vi "Interface Browser.vi"(5 "Caller Window Bounds":T1, 7 "Name (\"\" to Use Uuid)":string=".interface-browser", 10 "Init State (\"Macro: Initialize\")":string="Macro: Initialize") -> ()   [LabVIEW 2017]
uses:
  <vilib>/Utility/miscctls.llb/LVRectTypeDef.ctl
  Def-FilterOption.ctl
  <vilib>/Utility/miscctls.llb/LVPoint32TypeDef.ctl
  Def-TreeData.ctl
  <vilib>/Utility/miscctls.llb/LVPointTypeDef.ctl
  AdvanceAPI/CSM - Revert Arguments-Safe String.vi
  AdvanceAPI/CSM - Break Down Multiple States String.vi
  AdvanceAPI/CSM - Compact Multiple States.vi
  AdvanceAPI/CSM - Make String Arguments Safe.vi
  AdvanceAPI/CSM - Keywords.vi
  _Polymophic/Add State(s) to Queue By BOOL(Element).vi
  _csmHelper/API/Destroy.vi
  _csmHelper/API/Stop Undo.vi
  _csmHelper/API/Open Block Diagram.vi
  _csmHelper/API/Connect Paired Tunnels.vi
  _csmHelper/API/Add State Frame.vi
  _csmHelper/API/Start Undo.vi
  _csmHelper/API/Create From VI Reference.vi
  _csmHelper/API/Open Front Panel.vi
  _Polymophic/CSM - Filter Duplicated Lines.vi
  Communicable State Machine.lvlib
  _ui/csm-ui-support.lvlib
  _csmHelper/API with lvcsm Support/CSM-Helper API with lvcsm Support.lvlib
  _interfacebrowser/interfacebrowser.lvlib
  _csmHelper/CSM-Helper.lvclass
  _csmHelper/lvcsmFile/lvcsm File Support.lvlib
  _Shared/CSM Shared.lvlib
panel:
  in  "Option:All-CSM-VIs":bool
  in  "Scan Project":bool
  in  "Refresh":bool
  in  "Fast Forward":bool
  in  "Fast Reverse":bool
  in  "Skip to Beginning":bool
  in  "Skip to End":bool
  in  "Stop":bool
  in  "Play":bool
  in  "Open":bool
  in  "Option:Online Only":bool
  in  "Refresh lvcsm Cache":bool
  in  "Filter":string
  in  "FilterOption":T2
  in  "Reset Filter":bool
  in  "MainTree":string[](tree)
  in  "Option:Sync Filter On States":bool
  in  "Zoom Factor":dbl(slide)=0.1 min=0.1 max=1.0 step=0.001 scale=0.1..1.0
  in  "Interface-Filter":enum16{"API-Only", "UserDef States", "All"}(ring)=enum."UserDef States"
  in  "CSM-States":i32[](listbox) caption="Interface"
  in  "CSM-Status":i32[](listbox) caption="Status"
  out "StateInfo@Image":string
  out "Preview":picture
  out "String":string
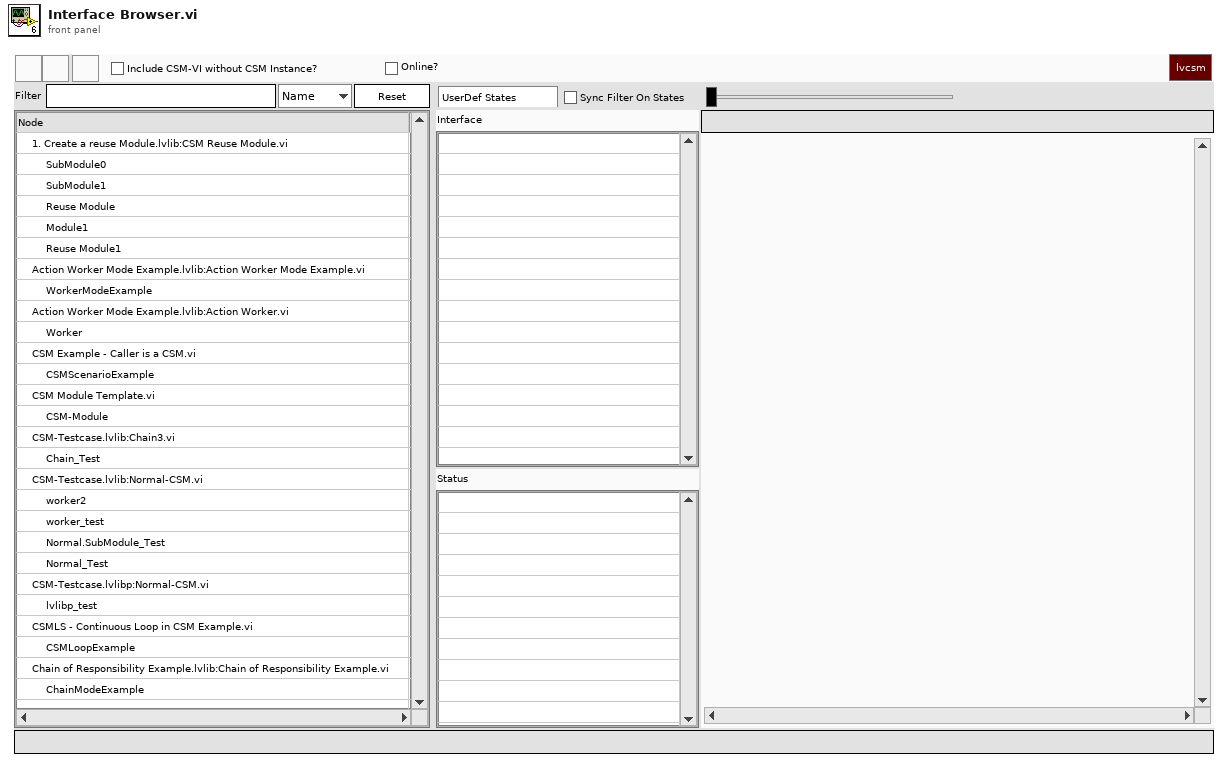
[diagram p1: front panel]
types:
  T1 = typedef "LVRectTypeDef.ctl" = cluster{"Left":i16, "Top":i16, "Right":i16, "Bottom":i16}
  T2 = typedef "Def-FilterOption.ctl" = enum16{"Name", "State"}
  T3 = enum32{"Invalid", "Standard", "Closed", "Hidden", "Minimized", "Maximized"}
  T4 = enum32{"invalid app kind", "Development System", "Run Time System", "Student Edition", "Embedded LabVIEW", "Evaluation", "Custom"}
  T5 = typedef "LVPointTypeDef.ctl" = cluster{"Horizontal":i16, "Vertical":i16}
  T6 = cluster{"Opton:All-CSM-VIs":bool, "Option:Online Only":bool}
  T7 = typedef "Communicable State Machine.lvlib/_CSM_Response Source Message.ctl" = cluster{"‘State":string, "’Arguments":string, "’Error":errorcluster}
  T8 = cluster{"Current VI Reference":refnum<vi>, "Close Panel on Exit?":bool}
  T9 = typedef "Def-TreeData.ctl" = cluster{"Type":string[], "Table":string[][]}
  T10 = cluster{"Core":cluster{"Current VI Reference":refnum<vi>, "Close Panel on Exit?":bool}, "BD-IMG":picture, "Tree":T9}
  T11 = typedef "LVPoint32TypeDef.ctl" = cluster{"Horizontal":i32, "Vertical":i32}
  T12 = cluster{"your data":bool, "PreviewMouseDown":bool, "PreviewMouseDownCoords":T11, "PreviewMouseDownOrigin":T11}
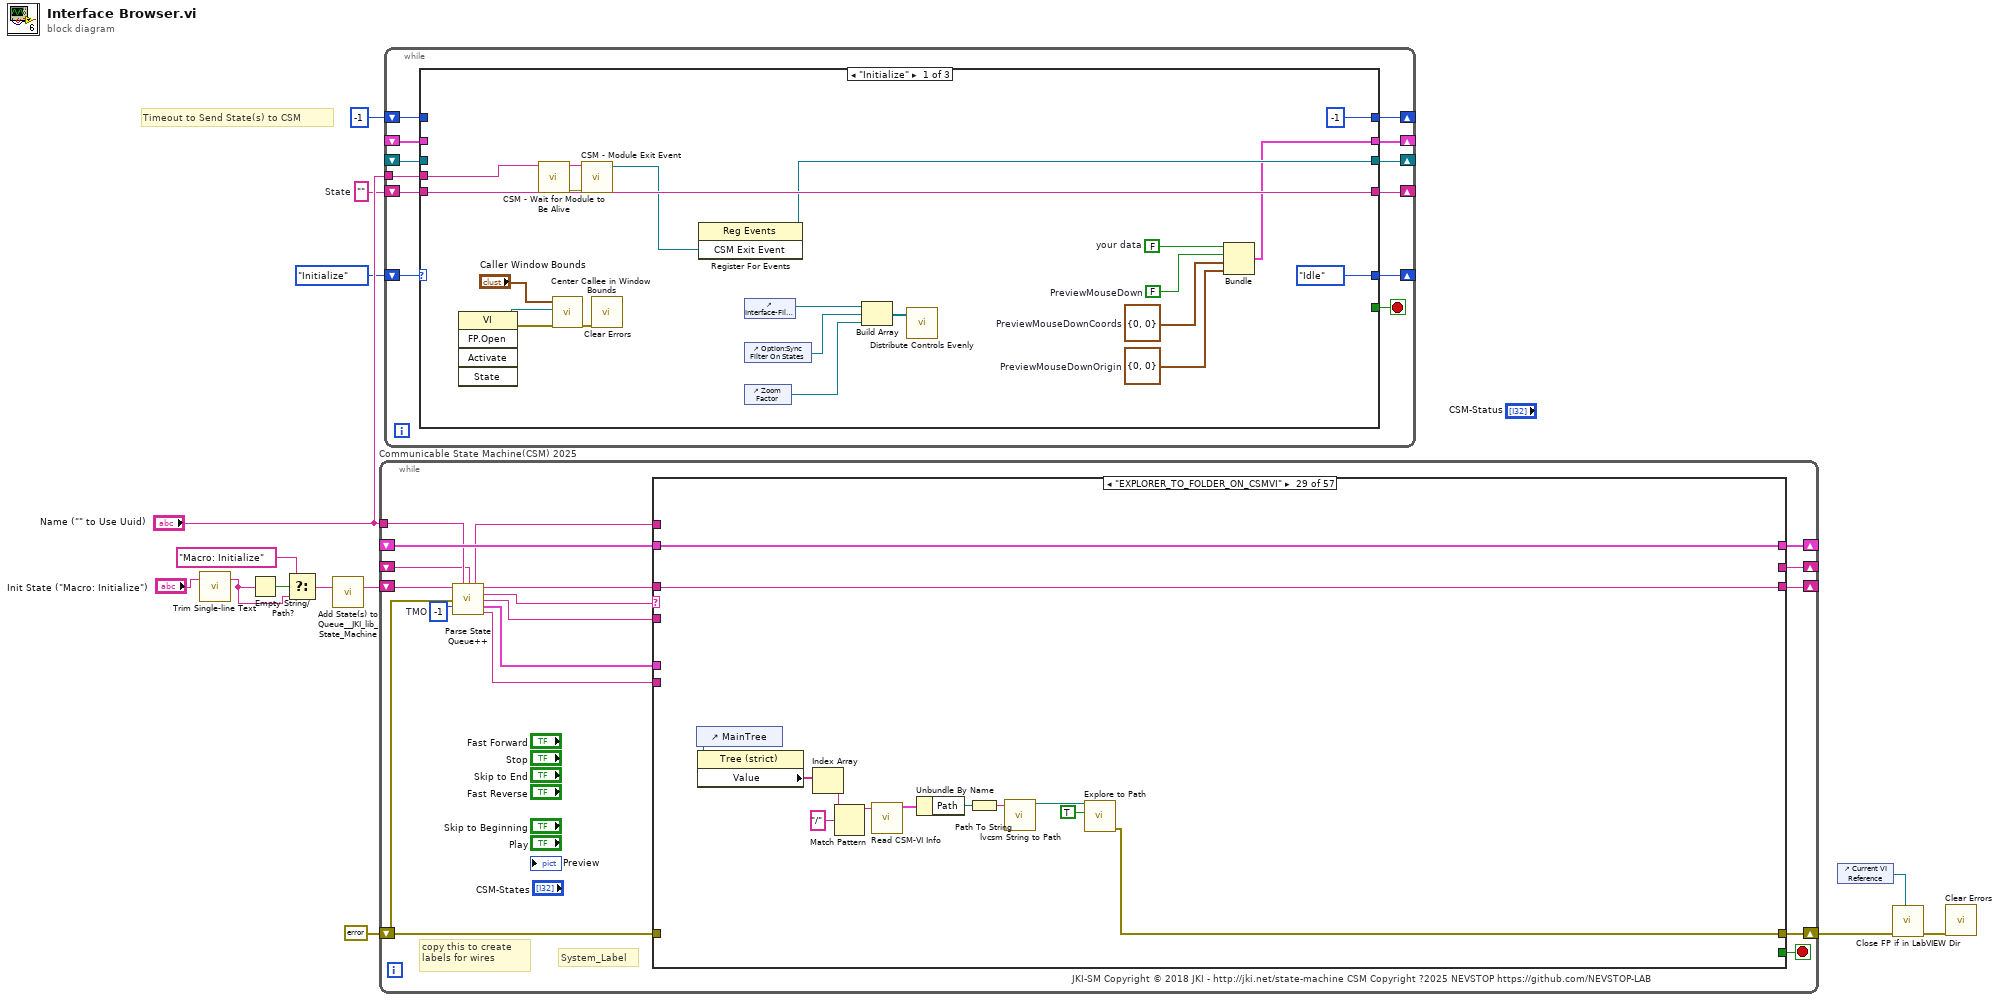
[diagram p0: block diagram]
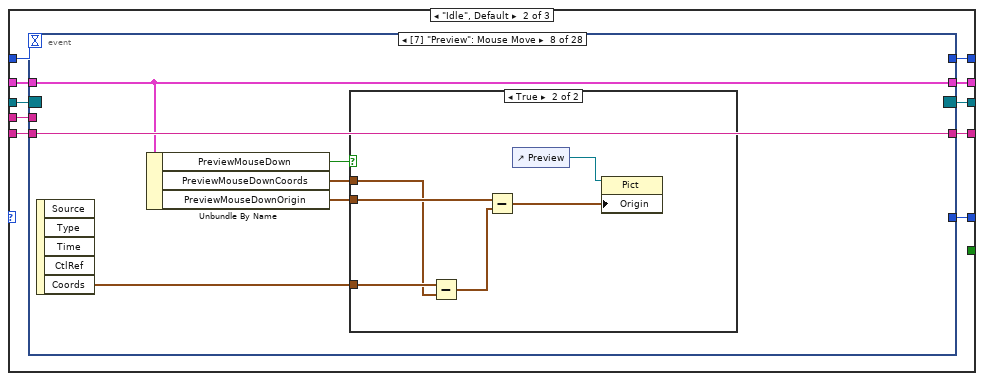
[diagram p2: hidden frame]
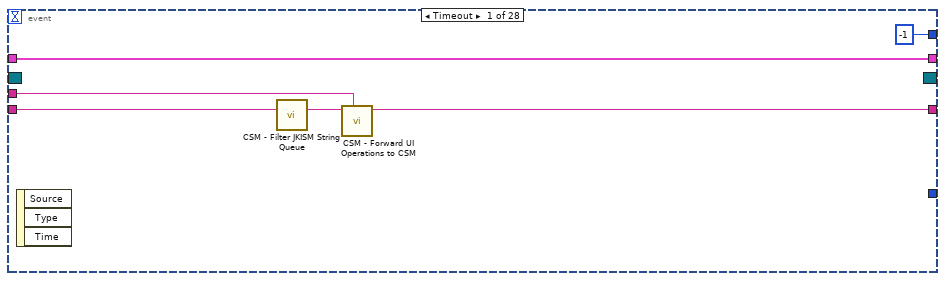
[diagram p3: hidden frame]
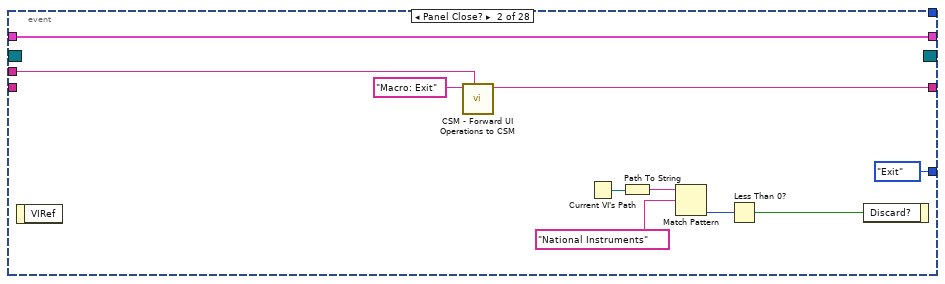
[diagram p4: hidden frame]
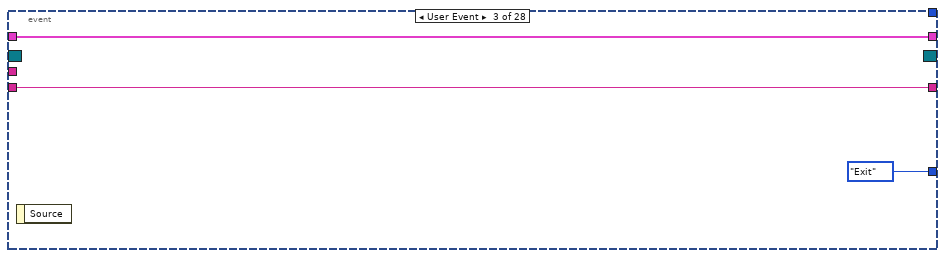
[diagram p5: hidden frame]
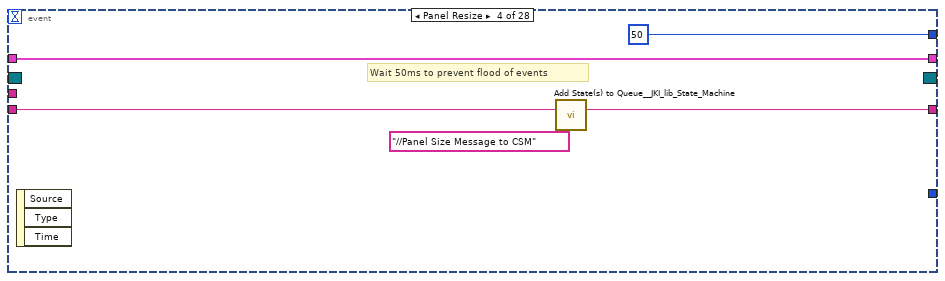
[diagram p6: hidden frame]
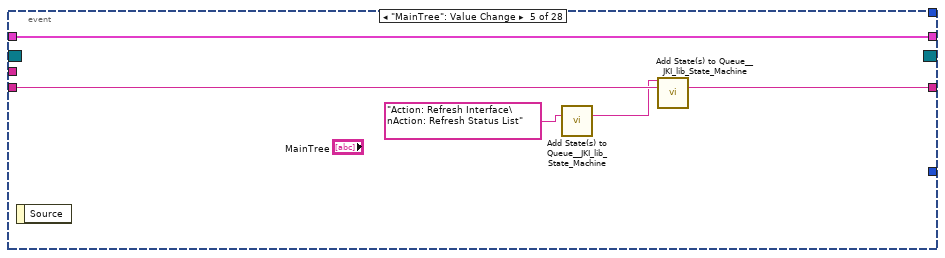
[diagram p7: hidden frame]
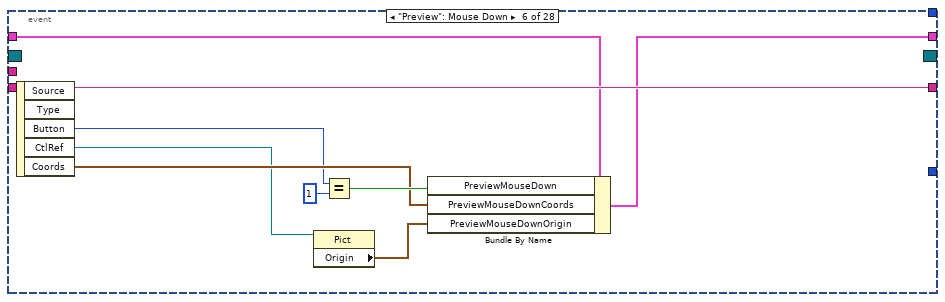
[diagram p8: hidden frame]
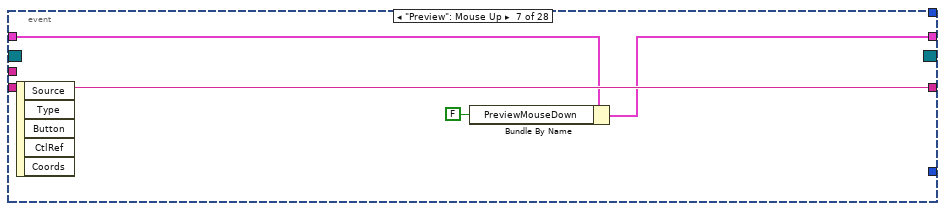
[diagram p9: hidden frame]
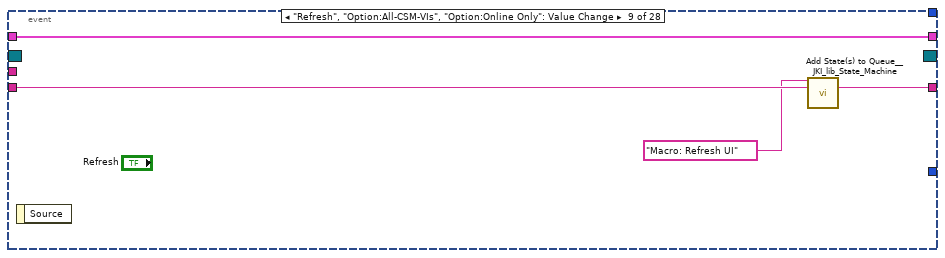
[diagram p11: hidden frame]
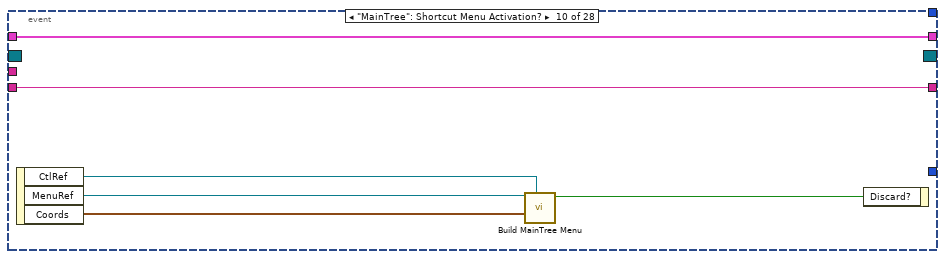
[diagram p12: hidden frame]
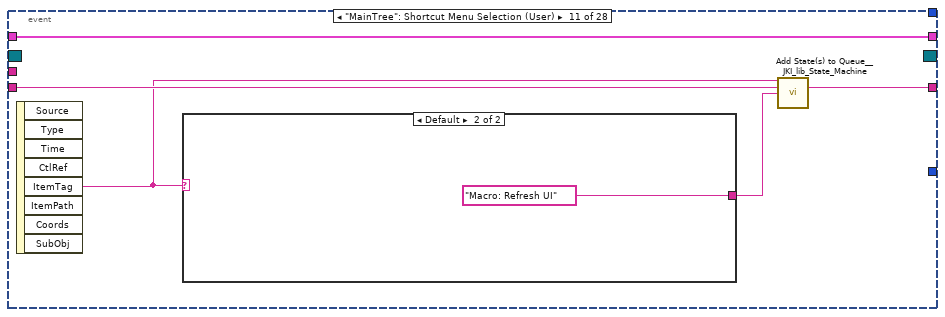
[diagram p13: hidden frame]
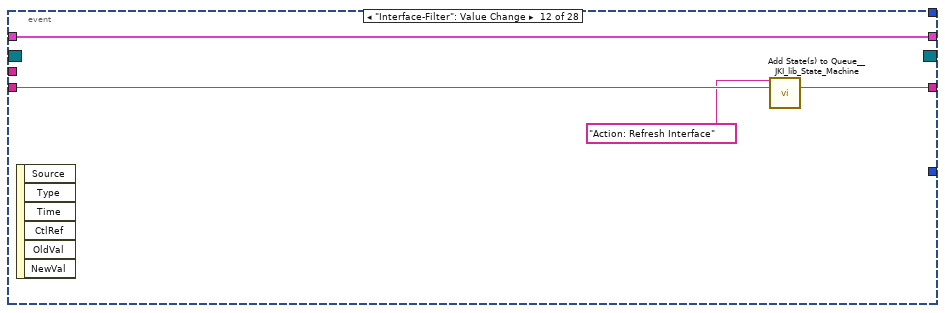
[diagram p15: hidden frame]
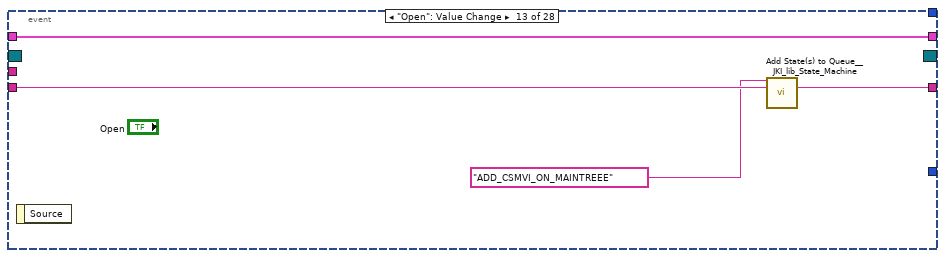
[diagram p16: hidden frame]
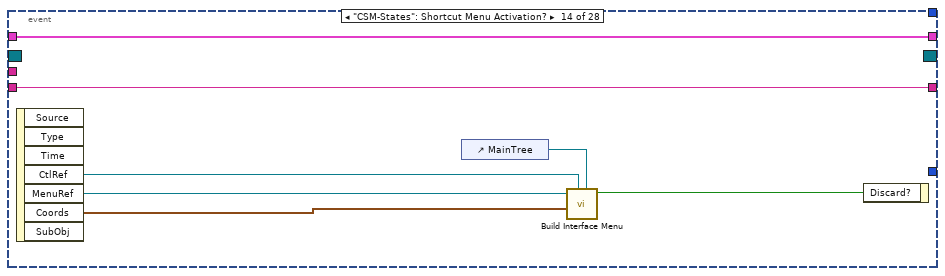
[diagram p17: hidden frame]
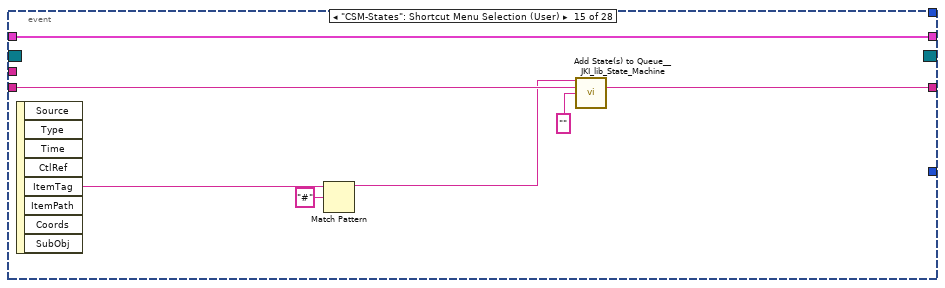
[diagram p18: hidden frame]
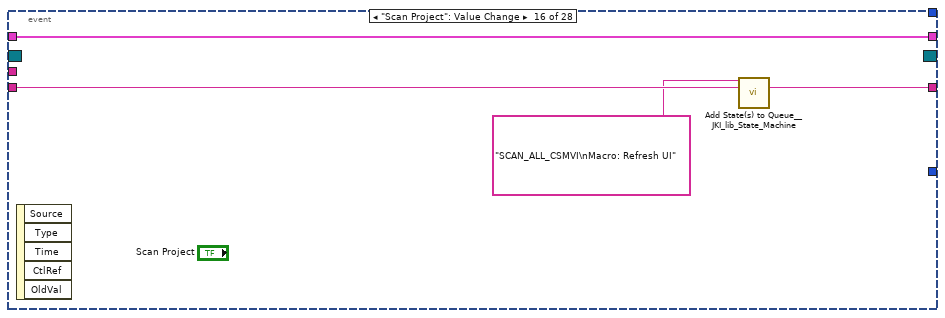
[diagram p19: hidden frame]
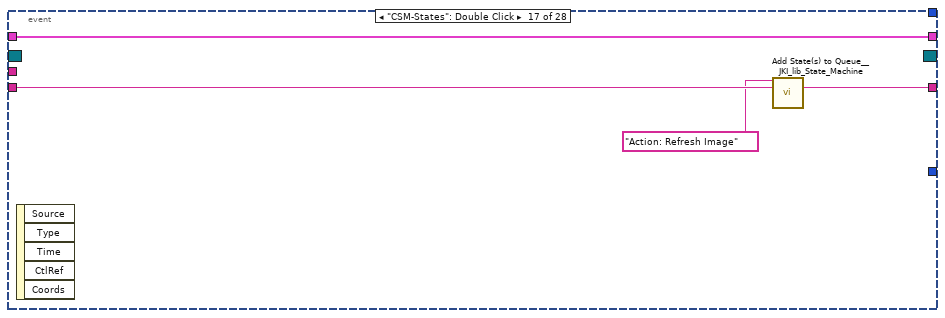
[diagram p20: hidden frame]
diagram:
  w12 = ""  # State
  # "Timeout to Send State(s) to CSM"
  n1 = call "Trim Single-line Text.vi"("single-line text"="Init State (\"Macro: Initialize\")") -> ("trimed text"=w5:string)  [unwired: 2 in]
  n2 = Empty String/Path?(string/path=w5) -> (empty?=w7:bool)
  n3 = Select(t="Macro: Initialize", s=w7, f=w5) -> (s? t:f=w6:string)
  n4 = call <vilib>:"Add State(s) to Queue__JKI_lib_State_Machine.vi"("State(s) in (\"\")"=w6) -> ("States Out"=w8:string)  [unwired: 14 in]
  n5 = while "Communicable State Machine(CSM) 2025" {
    shift-right: [w26] -> _
    shift-left: _ -> [w25]
    shift-right: [w29] -> w1
    shift-left: errorcluster {"status"=FALSE, "code"=0, "source"=""} ("error out") -> [w15]
    shift-right: [w28] -> _
    shift-left: w8 -> [w30]
    tunnel: "Name (\"\" to Use Uuid)" -> [w22]
    shift-right: [w23] -> _
    shift-left: _ -> [w17]
    stop <- w27 stop-if-true
    w24 = -1  # TMO
    # "JKI-SM Copyright © 2018 JKI - http://jki.net/state-machine CSM Copyright ?2025 NEVSTOP https://github.com/NEVSTOP-LAB"
    # "copy this to create labels for wires"
    # "System_Label"
    n6 = call "Parse State Queue++.vi"("State Queue"=w30, "Name (\"\" to Use UUID)"=w22, "Response Arguments"=w17, "Previous Error"=w15, "Dequeue (1 ms)"=w24) -> ("Name Used"=w16:string, "Remaining States"=w31:string, "Current State"=w18:string, "Arguments"=w19:string, "Additional Information"=w20:T7, "Source CSM"=w21:string)  [unwired: 5 in]
    n7 = case shown="\"EXPLORER_TO_FOLDER_ON_CSMVI\"" w18 {
      selector: w18 -> [_ _ _ w42 _ _ _ _ _ _ _ _ _ _ _ _ _ _ _ _ _ _ _ _ _ _ _ _ _ _ _ _ _ _ _ _ _ _ _ _ _ _ _ _ _ _ _ _ _ _ _ _ _ _ _ _ _]
      tunnel: w31 -> [w32 w35 w38 w46 w51 w57 w80 w86 w92 w102 w109 w121 w125 w128 w134 w149 w155 w158 w162 w166 w172 w174 w184 w198 w205 w222 w234 w255 w268 w281 w295 w309 w326 w328 w371 w396 w408 w420 w429 w450 w452 w457 w462 w474 w494 w506 w517 w528 w535 w551 w568 w607 w633 w648 w669 w689 w719]
      tunnel: w19 -> [_ _ _ _ _ w56 w76 w83 w89 w96 _ _ _ _ _ _ _ _ _ _ _ _ _ _ _ _ _ _ _ _ _ _ _ _ _ _ _ _ _ _ _ _ _ w470 w485 _ _ _ _ _ _ _ w629 _ _ _ w716]
      tunnel: w25 -> [w33 w34 w36 w44 w50 w62 w78 w84 w90 w100 w108 w115 w123 w126 _ w148 w150 w156 w160 w164 w170 w173 w183 w197 w208 w221 w233 w254 w267 w280 w294 w308 w325 w338 w376 w398 w410 w422 w428 w449 w454 w459 w461 w473 w493 w504 w515 w526 w536 w542 w566 w605 w632 w658 w678 w688 w718]
      tunnel: [_ _ _ w39 w52 errorcluster {"status"=FALSE, "code"=0, "source"=""} ("error out") w73 w81 w87 w103 _ _ _ _ _ _ w151 _ _ _ _ w175 w178 w193 _ w213 w226 w240 w257 w269 w283 w302 w324 w339 w375 w390 w404 w416 w427 w448 w455 w460 _ w464 w488 _ w508 _ w534 _ _ _ w631 _ _ w679 w720] -> w29
      tunnel: w15 -> [_ _ _ w40 w52 w60 w74 w82 w88 _ _ _ _ _ _ _ w152 _ _ _ _ w175 _ _ _ _ _ _ _ _ _ _ _ w339 _ _ _ _ _ _ w455 w460 _ _ _ _ _ _ _ _ _ _ _ _ _ _ w720]
      tunnel: [w32 w35 w37 w45 w51 w58 w79 w85 w91 w101 w109 w120 w124 w127 w133 w149 w154 w157 w161 w165 w171 w174 w184 w198 w206 w222 w234 w255 w268 w281 w295 w309 w326 w329 w372 w397 w409 w421 w429 w450 w453 w458 w462 w474 w494 w505 w516 w527 w537 w550 w567 w606 w633 w649 w670 w689 w719] -> w28
      tunnel: [_ _ _ _ _ _ TRUE _ _ _ _ _ TRUE _ _ _ _ _ _ _ _ _ _ _ _ _ _ _ _ _ _ _ _ _ _ _ _ _ _ _ _ _ _ _ _ _ _ _ _ _ _ _ _ _ _ _ _] -> w27
      tunnel: [w33 w34 w36 w44 w50 w62 w78 w84 w90 w99 w108 w119 w123 w126 w132 w148 w150 w156 w160 w164 w170 w173 w183 w197 w208 w221 w233 w254 w267 w280 w294 w308 w325 w338 w376 w398 w410 w422 w428 w449 w454 w459 w461 w473 w493 w504 w515 w525 w536 w542 w566 w605 w632 w658 w678 w688 w718] -> w26
      tunnel: w21 -> [_ _ _ _ _ w55 _ _ _ w97 _ _ _ _ _ _ _ _ _ _ _ _ _ _ _ _ _ _ _ _ _ _ _ _ _ _ _ _ w424 _ _ _ _ _ _ _ _ _ _ _ _ _ _ _ _ _ _]
      tunnel: w20 -> [_ _ _ _ _ w54 _ _ _ w98 _ _ _ _ _ _ _ _ _ _ _ _ _ _ _ _ _ _ _ _ _ _ _ _ _ _ _ _ _ _ _ _ _ _ _ _ _ _ _ _ _ _ _ _ _ _ _]
      tunnel: [_ _ _ "" w47 _ _ _ _ _ _ _ _ _ _ _ _ _ _ _ _ _ _ _ _ _ _ _ _ _ _ _ _ _ _ _ _ _ _ _ _ _ _ _ _ _ _ _ _ _ _ _ _ _ _ _ _] -> w23
      tunnel: w16 -> [_ _ _ w41 _ _ w75 _ _ _ _ _ _ _ _ _ _ _ _ _ _ _ _ _ _ _ _ _ _ _ _ _ _ _ _ _ _ _ _ _ _ _ _ _ _ _ _ _ w531 _ _ _ _ _ _ _ _]
      frame "", "Idle" {
      }
      frame "CSM Documentation" {
      }
      frame "---------- Core ----------" {
        n8 = call <vilib>:"Add State(s) to Queue__JKI_lib_State_Machine.vi"("State(s) in (\"\")"=w38) -> ("States Out"=w37:string)  [unwired: 14 in]
      }
      frame Default {
        n9 = call "CSM Unhandled State Error.vi"("error in (no error)"=w40, "Undefined State"=w42, "CSM Name"=w41) -> ("error out"=w39:errorcluster)  [unwired: 8 in]
        n10 = call <vilib>:"Add State(s) to Queue__JKI_lib_State_Machine.vi"("State(s) in (\"\")"=w46) -> ("States Out"=w45:string)  [unwired: 14 in]
      }
      frame "VI Reference" {
        n11 = Unbundle By Name(w50) -> ("Core"=w49:T8)
        n12 = Unbundle By Name(w49) -> ("Current VI Reference"=w48:refnum<vi>)
        n13 = call "CSM - Convert Data to HexStr.vi"("Variant"=w48) -> ("HEX String (0-9,A-F)"=w47:string)  [unwired: 8 in]
      }
      frame "Error Handler" {
        # "Clear error"
        n14 = case shown="Error" w60 {
          selector: w60 -> [_ w67]
          tunnel: [w66 w69] -> w59
          tunnel: w57 -> [w66 w68]
          tunnel: w56 -> [w65 _]
          tunnel: w55 -> [_ _]
          tunnel: w54 -> [_ _]
          tunnel: [w64 w67] -> w53
          frame No Error {
            n15 = call "CSM - Convert Argument to Error.vi"("Argument"=w65) -> ("Error"=w64:errorcluster)  [unwired: 4 in]
            n16 = flat-sequence {
              tunnel: w64 -> [_]
              frame #0 {
              }
            }
          }
          frame Error {
            n17 = call "CSM - Convert Error to Argument.vi"("Error"=w67) -> ("Argument"=w71:string)  [unwired: 4 in]
            n18 = call <vilib>:"Build State String with Arguments__JKI_lib_State_Machine.vi"("Arguments (\"\")"=w71, "State"="Error Occurred" ("Status with Arguments")) -> ("State with Arguments"=w70:string)  [unwired: 4 in]
            n19 = call "CSM - Broadcast Status Change.vi"("Status With Arguments"=w70, "State Queue"=w68) -> ("Remaining States"=w69:string)  [unwired: 13 in]
          }
        }
        n20 = call <vilib>:"Simple Error Handler.vi"("error in (no error)"=w53) -> ()  [unwired: 4 in, 5 out]
        n21 = call <vilib>:"Add State(s) to Queue__JKI_lib_State_Machine.vi"("State(s) in Front (\"\")"="// Post Error States", "State(s) in (\"\")"=w59) -> ("States Out"=w58:string)  [unwired: 13 in]
      }
      frame "Critical Error" {
        n22 = call "CSM Critical Error.vi"("error in (no error)"=w74, "Arugments (As Reason)"=w76, "CSM Name"=w75) -> ("error out"=w73:errorcluster)  [unwired: 8 in]
        n23 = call <vilib>:"Add State(s) to Queue__JKI_lib_State_Machine.vi"("State(s) in (\"\")"=w80) -> ("States Out"=w79:string)  [unwired: 14 in]
      }
      frame "Target Timeout Error" {
        n24 = call "CSM Target Timeout Error.vi"("error in (no error)"=w82, "Arguments (As CSM Name)"=w83) -> ("error out"=w81:errorcluster)  [unwired: 9 in]
        n25 = call <vilib>:"Add State(s) to Queue__JKI_lib_State_Machine.vi"("State(s) in (\"\")"=w86) -> ("States Out"=w85:string)  [unwired: 14 in]
      }
      frame "Target Error" {
        n26 = call "CSM Target Error.vi"("error in (no error)"=w88, "Arguments (As CSM Name)"=w89) -> ("error out"=w87:errorcluster)  [unwired: 9 in]
        n27 = call <vilib>:"Add State(s) to Queue__JKI_lib_State_Machine.vi"("State(s) in (\"\")"=w92) -> ("States Out"=w91:string)  [unwired: 14 in]
      }
      frame "Async Response", "Response" {
        n28 = Unbundle(w98) -> ("‘State"=w95:string, "’Arguments"=w94:string, "’Error"=w93:errorcluster)
        n29 = case shown="Default" w95 {
          tunnel: [w104] -> w101
          tunnel: w102 -> [w105]
          tunnel: [w107] -> w99
          tunnel: w100 -> [w107]
          tunnel: [w106] -> w103
          tunnel: w93 -> [w106]
          tunnel: w97 -> [_]
          tunnel: w96 -> [_]
          tunnel: w94 -> [_]
          frame Default {
            n30 = call <vilib>:"Add State(s) to Queue__JKI_lib_State_Machine.vi"("State(s) in (\"\")"=w105) -> ("States Out"=w104:string)  [unwired: 14 in]
          }
        }
      }
      frame "Async Message Posted" {
      }
      frame "Initialize Core Data" {
        # "originally closed?"
        # "exe?"
        # "If panel starts closed or is an EXE, then close it when we exit"
        n31 = control-ref of="Current VI Reference"() -> (w113:refnum<vi>)
        n32 = property class="VI"() -> ("FP.State"=w112:T3)  [unwired: 2 in, 2 out]
        n33 = property class="App"() -> ("App.Kind"=w118:T4)  [unwired: 2 in, 2 out]
        n34 = Equal?(x=w112, y=T3."Closed" ("Front Panel Window:State")) -> (x = y?=w110:bool)
        n35 = Equal?(x=w118, y=T4."Run Time System" ("Application:Kind")) -> (x = y?=w116:bool)
        n36 = Or(x=w110, y=w116) -> (x .or. y?=w114:bool)
        n37 = Bundle By Name(cluster=w115, "Core.Current VI Reference"=w113, "Core.Close Panel on Exit?"=w114) -> (w119:T10)
        n38 = call <vilib>:"Add State(s) to Queue__JKI_lib_State_Machine.vi"("State(s) in (\"\")"=w121) -> ("States Out"=w120:string)  [unwired: 14 in]
      }
      frame "Exit" {
        n39 = call <vilib>:"Add State(s) to Queue__JKI_lib_State_Machine.vi"("State(s) in (\"\")"=w125) -> ("States Out"=w124:string)  [unwired: 14 in]
      }
      frame "---------- Data ----------" {
        n40 = call <vilib>:"Add State(s) to Queue__JKI_lib_State_Machine.vi"("State(s) in (\"\")"=w128) -> ("States Out"=w127:string)  [unwired: 14 in]
      }
      frame "Data: Initialize" {
        w129 = T9 {"Type"=[], "Table"=[]}  # Tree
        w130 = picture data[5B]  # BD-IMG
        w131 = T8 {"Current VI Reference"=refnum, "Close Panel on Exit?"=FALSE}  # Core
        n41 = Bundle("Core"=w131, "BD-IMG"=w130, "Tree"=w129) -> (w132:T10)  [unwired: 1 in]
        n42 = call <vilib>:"Add State(s) to Queue__JKI_lib_State_Machine.vi"("State(s) in (\"\")"=w134) -> ("States Out"=w133:string)  [unwired: 14 in]
      }
      frame "Data: Update Indicators" {
        n43 = property class="App"() -> ("Project.ActiveProject"=w144:refnum<vi>)  [unwired: 2 in, 2 out]
        n44 = property class="Project"(reference=w144) -> ("Path"=w145:path)  [unwired: 1 in, 2 out]
        n45 = Strip Path(path=w145) -> (stripped path=w141:path)  [unwired: 1 out]
        n46 = local write "Preview"(picture data[5B] ("2D Picture 2")) -> ()
        n47 = local write "FilterOption"(Def-FilterOption."Name" ("FilterOption")) -> ()
        n48 = property on="Preview" class="Pict"("Origin"=T5 {"Horizontal"=0, "Vertical"=0}) -> ()  [unwired: 2 in, 2 out]
        n49 = Path To String(path=w141) -> (string=w140:string)
        n50 = call <vilib>:"Build State String with Arguments__JKI_lib_State_Machine.vi"("Arguments (\"\")"=w140, "State"="Interface Browser (CSM) ") -> ("State with Arguments"=w143:string)  [unwired: 4 in]
        n51 = property on="CSM-Status" class="LstBox (strict)"("Item Names"=string[] []) -> ()  [unwired: 2 in, 2 out]
        n52 = local write "Option:Sync Filter On States"(TRUE ("Option:Sync Filter On States")) -> ()
        n53 = local write "Zoom Factor"(0.7 ("Zoom Factor")) -> ()
        n54 = local write "Filter"("" ("Filter")) -> ()
        n55 = property class="VI"("Front Panel.Title"=w143) -> ()  [unwired: 2 in, 2 out]
      }
      frame "Data: Cleanup" {
        n56 = Unbundle By Name(w150) -> ("Core.Current VI Reference"=w153:refnum<vi>)
        n57 = Close Reference(reference=w153, error in (no error)=w152) -> (error out=w151:errorcluster)
        n58 = call <vilib>:"Add State(s) to Queue__JKI_lib_State_Machine.vi"("State(s) in (\"\")"=w155) -> ("States Out"=w154:string)  [unwired: 14 in]
      }
      frame "---------- Macro ----------" {
        n59 = call <vilib>:"Add State(s) to Queue__JKI_lib_State_Machine.vi"("State(s) in (\"\")"=w158) -> ("States Out"=w157:string)  [unwired: 14 in]
      }
      frame "Macro: Initialize" {
        n60 = call <vilib>:"Add State(s) to Queue__JKI_lib_State_Machine.vi"("State(s) in Front (\"\")"="Data: Initialize\nInitialize Core Data\nData: Update Indicators\nMacro: Refresh UI", "State(s) in (\"\")"=w162) -> ("States Out"=w161:string)  [unwired: 13 in]
      }
      frame "Macro: Refresh UI" {
        n61 = call <vilib>:"Add State(s) to Queue__JKI_lib_State_Machine.vi"("State(s) in Front (\"\")"="Action: Refresh(CSM-VI mode)\nAction: Refresh Symbol\nAction: Refresh Interface\nAction: Refresh Status List\nAction: Refresh Image\n", "State(s) in (\"\")"=w166) -> ("States Out"=w165:string)  [unwired: 13 in]
      }
      frame "Macro: Exit" {
        n62 = call <vilib>:"Add State(s) to Queue__JKI_lib_State_Machine.vi"("State(s) in Front (\"\")"="//Exit Sub-Modules ", "State(s) at Back (\"\")"="Data: Cleanup\nExit") -> ("States Out"=w168:string)  [unwired: 13 in]
        n63 = call <vilib>:"Add State(s) to Queue__JKI_lib_State_Machine.vi"("State(s) in Front (\"\")"=w168, "State(s) in (\"\")"=w172) -> ("States Out"=w171:string)  [unwired: 13 in]
      }
      frame "------ Menu Handler ------" {
      }
      frame "ADD_CSM_ON_CSMVI" {
        n64 = control-ref of="MainTree"() -> (w182:refnum<vi>)
        n65 = property class="Tree (strict)"(reference=w182) -> ("Value"=w181:string[])  [unwired: 1 in, 2 out]
        n66 = call "CSM Module Name"() -> ("CSM Module"=w179:string, "OK"=w177:bool)  [unwired: 17 in, 1 out]
        n67 = Index Array(array=w181) -> (element=w180:string)  [unwired: 1 in]
        n68 = call <vilib>:"Trim Whitespace.vi"("string"=w179) -> ("trimmed string"=w176:string)  [unwired: 1 in]
        n69 = case shown="True" w177 {
          tunnel: w180 -> [_ w187]
          tunnel: w176 -> [_ w186]
          tunnel: [_ w185] -> w178
          frame False {
          }
          frame True {
            n70 = call "Add CSM Module.vi"("CSM-VI"=w187, "CSM Name"=w186) -> ("error out"=w185:errorcluster)  [unwired: 9 in]
          }
        }
      }
      frame "ADD_CSM_ON_CSM" {
        n71 = control-ref of="MainTree"() -> (w196:refnum<vi>)
        n72 = property class="Tree (strict)"(reference=w196) -> ("Value"=w195:string[])  [unwired: 1 in, 2 out]
        n73 = Index Array(array=w195) -> (element=w190:string)  [unwired: 1 in]
        n74 = call "CSM Module Name2"() -> ("CSM Module"=w194:string, "OK"=w192:bool)  [unwired: 17 in, 1 out]
        n75 = Match Pattern(string=w190, regular expression="/") -> (before substring=w189:string)  [unwired: 1 in, 3 out]
        n76 = call <vilib>:"Trim Whitespace.vi"("string"=w194) -> ("trimmed string"=w191:string)  [unwired: 1 in]
        n77 = case shown="True" w192 {
          tunnel: w189 -> [_ w201]
          tunnel: w191 -> [_ w200]
          tunnel: [_ w199] -> w193
          frame False {
          }
          frame True {
            n78 = call "Add CSM Module.vi"("CSM-VI"=w201, "CSM Name"=w200) -> ("error out"=w199:errorcluster)  [unwired: 9 in]
          }
        }
      }
      frame "ADD_CSMVI_ON_MAINTREEE" {
        n79 = call "File Dialog"("pattern (all files)"="*.vi") -> ("selected path"=w203:path, "error out"=w204:errorcluster)  [unwired: 11 in, 2 out]
        n80 = case shown="Error" w204 {
          selector: w204 -> [w211 _]
          tunnel: w203 -> [w212 _]
          tunnel: ["Macro: Refresh UI" ("State(s) in Front (\"\")") _] -> w202
          frame No Error {
            n81 = call "Add CSM-VI.vi"("error in (no error)"=w211, "CSM-VI"=w212) -> ("error out"=w209:errorcluster)  [unwired: 9 in]
            n82 = call <vilib>:"Simple Error Handler.vi"("error in (no error)"=w209) -> ()  [unwired: 4 in, 5 out]
          }
          frame Error {
          }
        }
        n83 = call <vilib>:"Add State(s) to Queue__JKI_lib_State_Machine.vi"("State(s) in Front (\"\")"=w202, "State(s) in (\"\")"=w205) -> ("States Out"=w206:string)  [unwired: 13 in]
      }
      frame "RM_CSM_ON_CSM" {
        n84 = control-ref of="MainTree"() -> (w220:refnum<vi>)
        n85 = property class="Tree (strict)"(reference=w220) -> ("Value"=w219:string[])  [unwired: 1 in, 2 out]
        n86 = Index Array(array=w219) -> (element=w218:string)  [unwired: 1 in]
        n87 = Two Button Dialog(message="Are you sure to remove it?") -> (T button?=w214:bool)  [unwired: 2 in]
        n88 = Match Pattern(string=w218, regular expression="/") -> (after substring=w215:string)  [unwired: 1 in, 3 out]
        n89 = case shown="True" w214 {
          tunnel: w215 -> [_ w224]
          tunnel: [_ w223] -> w213
          frame False {
          }
          frame True {
            n90 = call "Delete CSM Module.vi"("CSM Name"=w224) -> ("error out"=w223:errorcluster)  [unwired: 10 in]
          }
        }
      }
      frame "RM_CSMVI_ON_CSMVI" {
        n91 = control-ref of="MainTree"() -> (w232:refnum<vi>)
        n92 = property class="Tree (strict)"(reference=w232) -> ("Value"=w231:string[])  [unwired: 1 in, 2 out]
        n93 = Index Array(array=w231) -> (element=w230:string)  [unwired: 1 in]
        n94 = Two Button Dialog(message="Are you sure to remove it?") -> (T button?=w227:bool)  [unwired: 2 in]
        n95 = Match Pattern(string=w230, regular expression="/") -> (before substring=w225:string)  [unwired: 1 in, 3 out]
        n96 = case shown="True" w227 {
          tunnel: w225 -> [_ w236]
          tunnel: [_ w235] -> w226
          frame False {
          }
          frame True {
            n97 = call "Delete CSM-VI.vi"("CSM Name"=w236) -> ("error out"=w235:errorcluster)  [unwired: 10 in]
          }
        }
      }
      frame "OPEN_CSMVI_ON_CSM", "OPEN_CSMVI_ON_CSMVI" {
        n98 = control-ref of="MainTree"() -> (w253:refnum<vi>)
        n99 = property class="Tree (strict)"(reference=w253) -> ("Value"=w252:string[])  [unwired: 1 in, 2 out]
        n100 = Index Array(array=w252) -> (element=w251:string)  [unwired: 1 in]
        n101 = Match Pattern(string=w251, regular expression="/") -> (before substring=w249:string)  [unwired: 1 in, 3 out]
        n102 = call "Read CSM-VI Info.vi"("CSM Name"=w249) -> ("Cluster 2"=w248:cluster{"Path":path})  [unwired: 9 in, 1 out]
        n103 = Unbundle By Name(w248) -> ("Path"=w238:path)
        n104 = Path To String(path=w238) -> (string=w237:string)
        n105 = call "lvcsm String to Path.vi"("Common Path"=w237) -> ("Path"=w239:path)  [unwired: 10 in]
        n106 = Open VI Reference(vi path=w239, options=2) -> (vi reference=w246:refnum<vi>, error out=w245:errorcluster)  [unwired: 4 in]
        n107 = call-poly "CSM-Helper API.vi"("error in (no error)"=w245, "VI"=w246) -> ("error out"=w243:errorcluster, "CSM-Helper.lvclass"=w244:refnum<class "CSM-Helper.lvclass">)  [unwired: 8 in]
        n108 = call-poly "CSM-Helper API.vi"("error in (no error)"=w243, "CSM-Helper in"=w244) -> ("error out"=w241:errorcluster, "CSM-Helper out"=w242:refnum<class "CSM-Helper.lvclass">)  [unwired: 8 in]
        n109 = call-poly "CSM-Helper API.vi"("error in (no error)"=w241, "CSM-Helper in"=w242) -> ("error out"=w240:errorcluster)  [unwired: 8 in, 1 out]
      }
      frame "EXPLORER_TO_FOLDER_ON_CSMVI" {
        n110 = control-ref of="MainTree"() -> (w266:refnum<vi>)
        n111 = property class="Tree (strict)"(reference=w266) -> ("Value"=w265:string[])  [unwired: 1 in, 2 out]
        n112 = Index Array(array=w265) -> (element=w264:string)  [unwired: 1 in]
        n113 = Match Pattern(string=w264, regular expression="/") -> (before substring=w262:string)  [unwired: 1 in, 3 out]
        n114 = call "Read CSM-VI Info.vi"("CSM Name"=w262) -> ("Cluster 2"=w261:cluster{"Path":path})  [unwired: 9 in, 1 out]
        n115 = Unbundle By Name(w261) -> ("Path"=w260:path)
        n116 = Path To String(path=w260) -> (string=w259:string)
        n117 = call "lvcsm String to Path.vi"("Common Path"=w259) -> ("Path"=w258:path)  [unwired: 10 in]
        n118 = call "Explore to Path.vi"("Select Directory? (F: Open Directory)"=TRUE, "Path"=w258) -> ("error out"=w257:errorcluster)  [unwired: 9 in]
      }
      frame "COPY_FULL_PATH_TO_CLIPBOARD" {
        n119 = control-ref of="MainTree"() -> (w279:refnum<vi>)
        n120 = property class="Tree (strict)"(reference=w279) -> ("Value"=w278:string[])  [unwired: 1 in, 2 out]
        n121 = Index Array(array=w278) -> (element=w277:string)  [unwired: 1 in]
        n122 = Match Pattern(string=w277, regular expression="/") -> (before substring=w275:string)  [unwired: 1 in, 3 out]
        n123 = call "Read CSM-VI Info.vi"("CSM Name"=w275) -> ("Cluster 2"=w274:cluster{"Path":path})  [unwired: 9 in, 1 out]
        n124 = Unbundle By Name(w274) -> ("Path"=w273:path)
        n125 = Path To String(path=w273) -> (string=w272:string)
        n126 = call "lvcsm String to Path.vi"("Common Path"=w272) -> ("Path"=w271:path)  [unwired: 10 in]
        n127 = Path To String(path=w271) -> (string=w270:string)
        n128 = invoke class="App" method="Clipboard.Write"("Param 0"=w270) -> (error out=w269:errorcluster)  [unwired: 3 in, 3 out]
      }
      frame "COPY_CNT_FOLDER_TO_CLIPBOARD" {
        n129 = control-ref of="MainTree"() -> (w293:refnum<vi>)
        n130 = property class="Tree (strict)"(reference=w293) -> ("Value"=w292:string[])  [unwired: 1 in, 2 out]
        n131 = Index Array(array=w292) -> (element=w291:string)  [unwired: 1 in]
        n132 = Match Pattern(string=w291, regular expression="/") -> (before substring=w289:string)  [unwired: 1 in, 3 out]
        n133 = call "Read CSM-VI Info.vi"("CSM Name"=w289) -> ("Cluster 2"=w288:cluster{"Path":path})  [unwired: 9 in, 1 out]
        n134 = Unbundle By Name(w288) -> ("Path"=w287:path)
        n135 = Path To String(path=w287) -> (string=w286:string)
        n136 = call "lvcsm String to Path.vi"("Common Path"=w286) -> ("Path"=w285:path)  [unwired: 10 in]
        n137 = Strip Path(path=w285) -> (stripped path=w282:path)  [unwired: 1 out]
        n138 = Path To String(path=w282) -> (string=w284:string)
        n139 = invoke class="App" method="Clipboard.Write"("Param 0"=w284) -> (error out=w283:errorcluster)  [unwired: 3 in, 3 out]
      }
      frame "GOTO_ON_CSMSTATE" {
        n140 = control-ref of="MainTree"() -> (w301:refnum<vi>)
        n141 = control-ref of="CSM-States"() -> (w306:refnum<vi>)
        n142 = property class="LstBox (strict)"(reference=w306) -> ("Item Names"=w307:string[], "Value"=w305:i32[])  [unwired: 1 in, 2 out]
        n143 = property class="Tree (strict)"(reference=w301) -> ("Value"=w300:string[])  [unwired: 1 in, 2 out]
        n144 = Index Array(array=w305) -> (element=w304:i32)  [unwired: 1 in]
        n145 = Index Array(array=w300) -> (element=w299:string)  [unwired: 1 in]
        n146 = Index Array(array=w307, index=w304) -> (element=w303:string)
        n147 = Match Pattern(string=w299, regular expression="/") -> (before substring=w297:string)  [unwired: 1 in, 3 out]
        n148 = call "Jump to CSM State.vi"("Type"=enum16{"CSM", "CSM-VI"}."CSM-VI", "State"=w303, "Name"=w297) -> ("error out"=w302:errorcluster)  [unwired: 8 in]
      }
      frame "GOTO_ON_CSMSTATUS" {
        (unwired) "@" ("string")
        n149 = control-ref of="CSM-Status"() -> (w314:refnum<vi>)
        n150 = property class="LstBox (strict)"(reference=w314) -> ("Item Names"=w317:string[], "Value"=w316:i32[])  [unwired: 1 in, 2 out]
        n151 = control-ref of="MainTree"() -> (w323:refnum<vi>)
        n152 = Index Array(array=w316) -> (element=w315:i32)  [unwired: 1 in]
        n153 = property class="Tree (strict)"(reference=w323) -> ("Value"=w322:string[])  [unwired: 1 in, 2 out]
        n154 = Index Array(array=w317, index=w315) -> (element=w313:string)
        n155 = Match Pattern(string=w313, regular expression="@") -> (after substring=w312:string)  [unwired: 1 in, 3 out]
        n156 = Index Array(array=w322) -> (element=w321:string)  [unwired: 1 in]
        n157 = call <vilib>:"Trim Whitespace.vi"("string"=w312) -> ("trimmed string"=w310:string)  [unwired: 1 in]
        n158 = Match Pattern(string=w321, regular expression="/") -> (before substring=w319:string)  [unwired: 1 in, 3 out]
        n159 = call "Jump to CSM State.vi"("Type"=enum16{"CSM", "CSM-VI"}."CSM-VI", "State"=w310, "Name"=w319) -> ("error out"=w324:errorcluster)  [unwired: 8 in]
      }
      frame "ADD_STATE_ON_CSMSTATE" {
        n160 = call "Add State"() -> ("State Name"=w337:string, "OK"=w330:bool, "error out"=w332:errorcluster)  [unwired: 17 in]
        n161 = Not(x=w332) -> (.not. x?=w333:bool)
        n162 = Empty String/Path?(string/path=w337) -> (empty?=w335:bool)
        n163 = And(x=w333, y=w330) -> (x .and. y?=w331:bool)
        n164 = Not(x=w335) -> (.not. x?=w336:bool)
        n165 = And(x=w336, y=w331) -> (x .and. y?=w334:bool)
        n166 = case shown="True" w334 {
          tunnel: w337 -> [_ w354]
          tunnel: [_ "RESCAN_INTERFACE_ON_CSMVI\nMacro: Refresh UI" ("State(s) in Front (\"\")")] -> w327
          frame False {
          }
          frame True {
            n167 = control-ref of="MainTree"() -> (w367:refnum<vi>)
            n168 = control-ref of="CSM-States"() -> (w368:refnum<vi>)
            n169 = property class="LstBox (strict)"(reference=w368) -> ("Item Names"=w369:string[])  [unwired: 1 in, 2 out]
            n170 = property class="Tree (strict)"(reference=w367) -> ("Value"=w366:string[])  [unwired: 1 in, 2 out]
            n171 = Index Array(array=w369) -> ()  [unwired: 1 in, 1 out]
            n172 = Index Array(array=w366) -> (element=w365:string)  [unwired: 1 in]
            n173 = Match Pattern(string=w365, regular expression="/") -> (before substring=w360:string)  [unwired: 1 in, 3 out]
            n174 = call "Read CSM-VI Info.vi"("CSM Name"=w360) -> ("error out"=w356:errorcluster, "Cluster 2"=w361:cluster{"Path":path})  [unwired: 9 in]
            n175 = Unbundle By Name(w361) -> ("Path"=w363:path)
            n176 = Path To String(path=w363) -> (string=w362:string)
            n177 = call "lvcsm String to Path.vi"("Common Path"=w362) -> ("Path"=w357:path)  [unwired: 10 in]
            n178 = Open VI Reference(vi path=w357, options=2, error in (no error)=w356) -> (vi reference=w358:refnum<vi>, error out=w359:errorcluster)  [unwired: 3 in]
            n179 = call-poly "CSM-Helper API.vi"("error in (no error)"=w359, "VI"=w358) -> ("error out"=w353:errorcluster, "CSM-Helper.lvclass"=w352:refnum<class "CSM-Helper.lvclass">)  [unwired: 8 in]
            n180 = call-poly "CSM-Helper API.vi"("error in (no error)"=w353, "CSM-Helper in"=w352) -> ("error out"=w351:errorcluster, "CSM-Helper out"=w350:refnum<class "CSM-Helper.lvclass">)  [unwired: 8 in]
            n181 = call-poly "CSM-Helper API.vi"("error in (no error)"=w351, "element"=w354, "CSM-Helper in"=w350) -> ("error out"=w343:errorcluster, "CSM-Helper out"=w342:refnum<class "CSM-Helper.lvclass">)  [unwired: 6 in, 1 out]
            n182 = call-poly "CSM-Helper API.vi"("error in (no error)"=w343, "CSM-Helper in"=w342) -> ("error out"=w340:errorcluster, "CSM-Helper out"=w341:refnum<class "CSM-Helper.lvclass">)  [unwired: 8 in]
            n183 = call-poly "CSM-Helper API.vi"("error in (no error)"=w340, "CSM-Helper in"=w341) -> ("error out"=w344:errorcluster, "CSM-Helper out"=w345:refnum<class "CSM-Helper.lvclass">)  [unwired: 8 in]
            n184 = call-poly "CSM-Helper API.vi"("error in (no error)"=w344, "CSM-Helper in"=w345) -> ("error out"=w349:errorcluster, "CSM-Helper out"=w348:refnum<class "CSM-Helper.lvclass">)  [unwired: 8 in]
            n185 = call-poly "CSM-Helper API.vi"("error in (no error)"=w349, "CSM-Helper in"=w348) -> ("error out"=w347:errorcluster)  [unwired: 8 in, 1 out]
            n186 = call <vilib>:"Simple Error Handler.vi"("error in (no error)"=w347) -> ()  [unwired: 4 in, 5 out]
          }
        }
        n187 = call <vilib>:"Add State(s) to Queue__JKI_lib_State_Machine.vi"("State(s) in Front (\"\")"=w327, "State(s) in (\"\")"=w328) -> ("States Out"=w329:string)  [unwired: 13 in]
      }
      frame "DELETE_STATE_ON_CSMSTATE" {
        n188 = Two Button Dialog(message="Are you sure?") -> (T button?=w373:bool)  [unwired: 2 in]
        n189 = case shown="True" w373 {
          tunnel: [_ w389] -> w375
          tunnel: [_ "RESCAN_INTERFACE_ON_CSMVI\nMacro: Refresh UI" ("State(s) in Front (\"\")")] -> w370
          frame False {
          }
          frame True {
            n190 = control-ref of="MainTree"() -> (w383:refnum<vi>)
            n191 = control-ref of="CSM-States"() -> (w387:refnum<vi>)
            n192 = property class="LstBox (strict)"(reference=w387) -> ("Item Names"=w388:string[], "Value"=w386:i32[])  [unwired: 1 in, 2 out]
            n193 = property class="Tree (strict)"(reference=w383) -> ("Value"=w382:string[])  [unwired: 1 in, 2 out]
            n194 = Index Array(array=w386) -> (element=w385:i32)  [unwired: 1 in]
            n195 = Index Array(array=w382) -> (element=w381:string)  [unwired: 1 in]
            n196 = Index Array(array=w388, index=w385) -> (element=w384:string)
            n197 = Match Pattern(string=w381, regular expression="/") -> (before substring=w379:string)  [unwired: 1 in, 3 out]
            n198 = call "Delete CSM State.vi"("Type"=enum16{"CSM", "CSM-VI"}."CSM-VI", "State"=w384, "Name"=w379) -> ("Error Out"=w389:errorcluster)  [unwired: 8 in]
          }
        }
        n199 = call <vilib>:"Add State(s) to Queue__JKI_lib_State_Machine.vi"("State(s) in Front (\"\")"=w370, "State(s) in (\"\")"=w371) -> ("States Out"=w372:string)  [unwired: 13 in]
      }
      frame "COPY_TO_CLIPBOARD_ON_CSMSTATE" {
        n200 = control-ref of="CSM-States"() -> (w394:refnum<vi>)
        n201 = property class="LstBox (strict)"(reference=w394) -> ("Item Names"=w395:string[], "Value"=w393:i32[])  [unwired: 1 in, 2 out]
        n202 = Index Array(array=w393) -> (element=w392:i32)  [unwired: 1 in]
        n203 = Index Array(array=w395, index=w392) -> (element=w391:string)
        n204 = invoke class="App" method="Clipboard.Write"("Param 0"=w391) -> (error out=w390:errorcluster)  [unwired: 3 in, 3 out]
        n205 = call <vilib>:"Add State(s) to Queue__JKI_lib_State_Machine.vi"("State(s) in (\"\")"=w396) -> ("States Out"=w397:string)  [unwired: 14 in]
      }
      frame "COPY_STATUS_TO_CLIPBOARD_ON_CSMSTATUS" {
        n206 = control-ref of="CSM-Status"() -> (w403:refnum<vi>)
        n207 = property class="LstBox (strict)"(reference=w403) -> ("Item Names"=w407:string[], "Value"=w406:i32[])  [unwired: 1 in, 2 out]
        n208 = Index Array(array=w406) -> (element=w405:i32)  [unwired: 1 in]
        n209 = Index Array(array=w407, index=w405) -> (element=w402:string)
        n210 = Match Pattern(string=w402, regular expression="@") -> (before substring=w400:string)  [unwired: 1 in, 3 out]
        n211 = call <vilib>:"Trim Whitespace.vi"("string"=w400) -> ("trimmed string"=w399:string)  [unwired: 1 in]
        n212 = invoke class="App" method="Clipboard.Write"("Param 0"=w399) -> (error out=w404:errorcluster)  [unwired: 3 in, 3 out]
        n213 = call <vilib>:"Add State(s) to Queue__JKI_lib_State_Machine.vi"("State(s) in (\"\")"=w408) -> ("States Out"=w409:string)  [unwired: 14 in]
      }
      frame "COPY_STATE_TO_CLIPBOARD_ON_CSMSTATUS" {
        n214 = control-ref of="CSM-Status"() -> (w415:refnum<vi>)
        n215 = property class="LstBox (strict)"(reference=w415) -> ("Item Names"=w419:string[], "Value"=w418:i32[])  [unwired: 1 in, 2 out]
        n216 = Index Array(array=w418) -> (element=w417:i32)  [unwired: 1 in]
        n217 = Index Array(array=w419, index=w417) -> (element=w414:string)
        n218 = Match Pattern(string=w414, regular expression="@") -> (after substring=w412:string)  [unwired: 1 in, 3 out]
        n219 = call <vilib>:"Trim Whitespace.vi"("string"=w412) -> ("trimmed string"=w411:string)  [unwired: 1 in]
        n220 = invoke class="App" method="Clipboard.Write"("Param 0"=w411) -> (error out=w416:errorcluster)  [unwired: 3 in, 3 out]
        n221 = call <vilib>:"Add State(s) to Queue__JKI_lib_State_Machine.vi"("State(s) in (\"\")"=w420) -> ("States Out"=w421:string)  [unwired: 14 in]
      }
      frame "SCAN_ALL_CSMVI" {
        n222 = case shown="\"\"" w424 {
          selector: w424 -> [w431 _]
          tunnel: [w430 w432] -> w423
          frame Default {
            n223 = call "lvcsm String to Path.vi"("Common Path"=w431) -> ("Path"=w430:path)  [unwired: 10 in]
          }
          frame "" {
            n224 = property class="App"() -> ("Project.ActiveProject"=w434:refnum<vi>)  [unwired: 2 in, 2 out]
            n225 = property class="Project"(reference=w434) -> ("Path"=w433:path)  [unwired: 1 in, 2 out]
            n226 = Strip Path(path=w433) -> (stripped path=w432:path)  [unwired: 1 out]
          }
        }
        n227 = Two Button Dialog(message="Scan for CSM Modules?") -> (T button?=w425:bool)  [unwired: 2 in]
        n228 = case shown="True" w425 {
          tunnel: [_ w437] -> w427
          tunnel: w423 -> [_ w436]
          frame False {
          }
          frame True {
            n229 = property class="VI"() -> ("Front Panel.PanelBounds"=w435:T1)  [unwired: 2 in, 2 out]
            n230 = call "Scan CSM-VI.vi"("Block Diagram Window:Window Bounds"=w435, "Root"=w436) -> ("Error Out"=w437:errorcluster)  [unwired: 9 in]
          }
        }
      }
      frame "RESCAN_INTERFACE_ON_CSMVI" {
        n231 = control-ref of="MainTree"() -> (w447:refnum<vi>)
        n232 = property class="Tree (strict)"(reference=w447) -> ("Value"=w446:string[])  [unwired: 1 in, 2 out]
        n233 = Index Array(array=w446) -> (element=w445:string)  [unwired: 1 in]
        n234 = Match Pattern(string=w445, regular expression="/") -> (before substring=w443:string)  [unwired: 1 in, 3 out]
        n235 = call "Read CSM-VI Info.vi"("CSM Name"=w443) -> ("error out"=w438:errorcluster, "Cluster 2"=w442:cluster{"Path":path})  [unwired: 9 in]
        n236 = Unbundle By Name(w442) -> ("Path"=w440:path)
        n237 = Path To String(path=w440) -> (string=w441:string)
        n238 = call "lvcsm String to Path.vi"("Common Path"=w441) -> ("Path"=w439:path)  [unwired: 10 in]
        n239 = call "Add CSM-VI.vi"("error in (no error)"=w438, "CSM-VI"=w439) -> ("error out"=w448:errorcluster)  [unwired: 9 in]
      }
      frame "CODEPREVIEW_ON_CSMSTATE" {
        n240 = call <vilib>:"Add State(s) to Queue__jki_lib_state_machine.vi"("State(s) in Front (\"\")"="Action: Refresh Image" ("State(s) in Front (\"\")"), "State(s) in (\"\")"=w452) -> ("States Out"=w453:string)  [unwired: 13 in]
      }
      frame "CODEPREVIEW_ON_CSMSTATUS" {
        n241 = call <vilib>:"Add State(s) to Queue__jki_lib_state_machine.vi"("State(s) in Front (\"\")"="Action: Refresh Image2" ("State(s) in Front (\"\")"), "State(s) in (\"\")"=w457) -> ("States Out"=w458:string)  [unwired: 13 in]
      }
      frame "---------- API ----------" {
      }
      frame "API: Set Current CSMVI" {
        n242 = control-ref of="MainTree"() -> (w472:refnum<vi>)
        n243 = property class="Tree (strict)"(reference=w472) -> (reference out=w466:refnum<vi>, error out=w465:errorcluster, "All Tags"=w471:string[])  [unwired: 1 in]
        n244 = for {
          tunnel: w471 -> [w482] mode=indexing
          tunnel: [w482] -> w468 mode=indexing if=w480
          n245 = Match Pattern(string=w482, regular expression="/") -> (offset past match=w481:i32)  [unwired: 1 in, 3 out]
          n246 = Less Than 0?(x=w481) -> (x < 0?=w480:bool)
        }
        n247 = for {
          tunnel: w468 -> [w479] mode=indexing
          tunnel: w470 -> [w478]
          tunnel: [w477] -> w469 if=w475
          i -> [w477]
          stop <- w475 stop-if-true
          n248 = Search/Split String(string=w479, search string/char (-)=w478) -> (offset of match=w476:i32)  [unwired: 1 in, 2 out]
          n249 = Greater Or Equal To 0?(x=w476) -> (x >= 0?=w475:bool)
        }
        n250 = Index Array(array=w468, index=w469) -> (element=w467:string)
        n251 = Build Array(w467) -> (w463:string[])
        n252 = property class="Tree (strict)"(reference=w466, error in=w465, "Value"=w463) -> (error out=w464:errorcluster)  [unwired: 1 out]
      }
      frame "API: Set Current CSM" {
        n253 = control-ref of="MainTree"() -> (w492:refnum<vi>)
        n254 = property class="Tree (strict)"(reference=w492) -> (reference out=w490:refnum<vi>, error out=w489:errorcluster, "All Tags"=w486:string[])  [unwired: 1 in]
        n255 = for {
          tunnel: w486 -> [w502] mode=indexing
          tunnel: w485 -> [w499]
          tunnel: [w496] -> w484 if=w495
          i -> [w496]
          stop <- w495 stop-if-true
          n256 = Match Pattern(string=w502, regular expression="/") -> (after substring=w500:string, offset past match=w501:i32)  [unwired: 1 in, 2 out]
          n257 = Equal?(x=w500, y=w499) -> (x = y?=w498:bool)
          n258 = Greater Or Equal To 0?(x=w501) -> (x >= 0?=w497:bool)
          n259 = And(x=w498, y=w497) -> (x .and. y?=w495:bool)
        }
        n260 = Index Array(array=w486, index=w484) -> (element=w491:string)
        n261 = Build Array(w491) -> (w487:string[])
        n262 = property class="Tree (strict)"(reference=w490, error in=w489, "Value"=w487) -> (error out=w488:errorcluster)  [unwired: 1 out]
      }
      frame "---------- Action ----------" {
        n263 = call <vilib>:"Add State(s) to Queue__JKI_lib_State_Machine.vi"("State(s) in (\"\")"=w506) -> ("States Out"=w505:string)  [unwired: 14 in]
      }
      frame "Action: Refresh(CSM mode)" {
        n264 = control-ref of="MainTree"() -> (w514:refnum<vi>)
        n265 = call "build tree table in CSM mode.vi"() -> ("Error Out"=w508:errorcluster, "Type"=w509:string[], "Tree Table"=w510:string[][])  [unwired: 9 in]
        n266 = call "Populate Tree with Delimited Strings_csm.vi"("Default Symbol"=0, "Delimiter"="/", "Items (Delimited)"=w510, "Tree Control"=w514) -> ("error out"=w512:errorcluster, "Tree Control Dup"=w511:refnum<vi>)  [unwired: 5 in, 1 out]
        n267 = property class="Tree"(reference=w511, error in=w512, "RowHdrs[]"=w509) -> ()  [unwired: 2 out]
        n268 = call <vilib>:"Add State(s) to Queue__JKI_lib_State_Machine.vi"("State(s) in (\"\")"=w517) -> ("States Out"=w516:string)  [unwired: 14 in]
      }
      frame "Action: Refresh(CSM-VI mode)" {
        n269 = Bundle By Name(cluster=T6 {"Opton:All-CSM-VIs"=FALSE, "Option:Online Only"=FALSE} ("Option"), "Opton:All-CSM-VIs"="Option:All-CSM-VIs", "Option:Online Only"="Option:Online Only") -> (w520:T6)
        n270 = call "build tree table in CSM-VI mode.vi"("Option"=w520) -> ("Type"=w523:string[], "Tree Table"=w524:string[][])  [unwired: 8 in, 1 out]
        n271 = Bundle By Name(cluster=w526, "Tree.Table"=w524, "Tree.Type"=w523) -> (w525:T10)
        n272 = call <vilib>:"Add State(s) to Queue__JKI_lib_State_Machine.vi"("State(s) in Front (\"\")"="Action: Update Tree" ("State(s) in Front (\"\")"), "State(s) in (\"\")"=w528) -> ("States Out"=w527:string)  [unwired: 13 in]
      }
      frame "Action: Update Online CSMs" {
        n273 = call "Refresh Online CSMs in lvcsm.vi"("Caller"=w531) -> ("error out"=w530:errorcluster, "Array W/ Subset Deleted"=w529:string[])  [unwired: 9 in]
        n274 = Empty Array?(array=w529) -> (empty?=w533:bool)
        n275 = Merge Errors(w530) -> (w534:errorcluster)
        n276 = call-poly "Add State(s) to Queue By BOOL++.vi"("FALSE (\"\")"="Action: Refresh(CSM-VI mode)" ("State(s) in Front (\"\")"), "Condition"=w533, "State Queue (\"\")"=w535) -> ("Remaining States"=w537:string)  [unwired: 8 in]
      }
      frame "Action: Update Tree" {
        n277 = Unbundle By Name(w542) -> ("Tree"=w541:T9)
        n278 = call "Filter Tree Data.vi"("FilterOption"="FilterOption", "Filter"="Filter", "TreeData"=w541) -> ("TreeData 2"=w543:T9)  [unwired: 8 in]
        n279 = Unbundle By Name(w543) -> ("Table"=w539:string[][], "Type"=w538:string[])
        n280 = control-ref of="MainTree"() -> (w549:refnum<vi>)
        n281 = call "Populate Tree with Delimited Strings_csm.vi"("Default Symbol"=0, "Delimiter"="/", "Items (Delimited)"=w539, "Tree Control"=w549) -> ("error out"=w547:errorcluster, "Tree Control Dup"=w546:refnum<vi>)  [unwired: 5 in, 1 out]
        n282 = property class="Tree"(reference=w546, error in=w547, "RowHdrs[]"=w538) -> ()  [unwired: 2 out]
        n283 = call <vilib>:"Add State(s) to Queue__JKI_lib_State_Machine.vi"("State(s) in (\"\")"=w551) -> ("States Out"=w550:string)  [unwired: 14 in]
      }
      frame "Action: Refresh Interface" {
        n284 = control-ref of="MainTree"() -> (w558:refnum<vi>)
        n285 = property class="Tree (strict)"(reference=w558) -> ("Value"=w557:string[])  [unwired: 1 in, 2 out]
        n286 = for {
          tunnel: [w596] -> w565 mode=indexing
          tunnel: w557 -> [w594] mode=indexing
          n287 = Match Pattern(string=w594, regular expression="/") -> (before substring=w593:string)  [unwired: 1 in, 3 out]
          n288 = call "Read CSM States By CSM-VI.vi"("CSM VI"=w593) -> ("Array"=w597:string[])  [unwired: 9 in, 1 out]
          n289 = Bundle("Array"=w597) -> (w596:cluster{"Array":string[]})  [unwired: 1 in]
        }
        n290 = Delete From Array(array=w565, index=0) -> (deleted portion=w562:cluster{"Array":string[]}, array with subset deleted=w563:cluster{"Array":string[]}[])  [unwired: 1 in]
        n291 = Unbundle(w562) -> ("Array"=w561:string[])
        n292 = for {
          tunnel: w563 -> [w589] mode=indexing
          shift-right: [w584] -> w560
          shift-left: w561 -> [w588]
          n293 = Unbundle(w589) -> ("Array"=w587:string[])
          n294 = Build Array (concatenate)(w588, w587) -> (w585:string[])
          n295 = call "_Remove Duplicates Strings.vi"("Input Array"=w585) -> ("Indices of Removed Elements"=w586:i32[])  [unwired: 1 out]
          n296 = for {
            tunnel: w586 -> [w591] mode=indexing
            tunnel: w585 -> [w592]
            tunnel: [w590] -> w584 mode=indexing
            n297 = Index Array(array=w592, index=w591) -> (element=w590:string)
          }
        }
        n298 = local read "FilterOption"() -> (w554:T2)
        n299 = local read "Filter"() -> (w553:string)
        n300 = call "filter CSM States.vi"("Interface-Filter"="Interface-Filter", "Array"=w560) -> ("filtered array"=w555:string[])  [unwired: 9 in]
        n301 = call <vilib>:"Add State(s) to Queue__JKI_lib_State_Machine.vi"("State(s) in (\"\")"=w568) -> ("States Out"=w567:string)  [unwired: 14 in]
        n302 = case shown="\"State\"" w554 {
          tunnel: [w569 w573] -> w556
          tunnel: w555 -> [w569 w572]
          tunnel: w553 -> [_ w571]
          tunnel: "Option:Sync Filter On States" -> [_ w570]
          frame "Name", Default {
          }
          frame "State" {
            n303 = case shown="False" w570 {
              tunnel: [w574 w577] -> w573
              tunnel: w572 -> [w574 w576]
              tunnel: w571 -> [_ w575]
              frame False {
              }
              frame True {
                n304 = for {
                  tunnel: [w580] -> w577 mode=indexing if=w578
                  tunnel: w576 -> [w580] mode=indexing
                  tunnel: w575 -> [w579]
                  n305 = To Lower Case(string=w579) -> (all lower case string=w581:string)
                  n306 = To Lower Case(string=w580) -> (all lower case string=w582:string)
                  n307 = Match Pattern(string=w582, regular expression=w581) -> (offset past match=w583:i32)  [unwired: 1 in, 3 out]
                  n308 = Greater Or Equal To 0?(x=w583) -> (x >= 0?=w578:bool)
                }
              }
            }
          }
        }
        n309 = property on="CSM-States" class="LstBox (strict)"("Item Names"=w556) -> ()  [unwired: 2 in, 2 out]
      }
      frame "Action: Refresh Status List" {
        n310 = control-ref of="MainTree"() -> (w604:refnum<vi>)
        n311 = property class="Tree (strict)"(reference=w604) -> ("Value"=w603:string[])  [unwired: 1 in, 2 out]
        n312 = Index Array(array=w603) -> (element=w602:string)  [unwired: 1 in]
        n313 = Match Pattern(string=w602, regular expression="/") -> (before substring=w600:string)  [unwired: 1 in, 3 out]
        n314 = call "Read CSM Status By CSM-VI.vi"("CSM VI"=w600) -> ("Array 3"=w599:cluster{"Status":string, "InState":string}[])  [unwired: 9 in, 1 out]
        n315 = disable-structure shown="Enabled" {
          disable-tunnel: w599 -> [w610 w615 _]
          disable-tunnel: [w608 w613 _] -> w598
          frame Disabled {
            n316 = for {
              tunnel: w610 -> [w612] mode=indexing
              tunnel: [w611] -> w609 mode=indexing
              n317 = Unbundle(w612) -> ("Status"=w611:string)  [unwired: 1 out]
            }
            n318 = call "_Remove Duplicates Strings.vi"("Input Array"=w609) -> ("Output Array"=w608:string[])  [unwired: 1 out]
          }
          frame Enabled {
            n319 = for {
              tunnel: w615 -> [w619] mode=indexing
              tunnel: [w617] -> w614 mode=indexing
              n320 = Unbundle(w619) -> ("Status"=w618:string, "InState"=w616:string)
              n321 = case shown="\"\"" w616 {
                selector: w616 -> [w621 _]
                tunnel: w618 -> [w623 w624]
                tunnel: [w622 w624] -> w617
                frame Default {
                  n322 = Concatenate Strings(w623, " @ " ("string"), w621) -> (w622:string)
                }
                frame "" {
                }
              }
            }
            n323 = call "_Remove Duplicates Strings.vi"("Input Array"=w614) -> ("Output Array"=w613:string[])  [unwired: 1 out]
          }
          frame Disabled {
          }
        }
        n324 = call <vilib>:"Add State(s) to Queue__JKI_lib_State_Machine.vi"("State(s) in (\"\")"=w607) -> ("States Out"=w606:string)  [unwired: 14 in]
        n325 = property on="CSM-Status" class="LstBox (strict)"("Item Names"=w598) -> ()  [unwired: 2 in, 2 out]
      }
      frame "Action: Refresh Image API" {
        n326 = Match Pattern(string=w629, regular expression="@") -> (before substring=w627:string, after substring=w626:string)  [unwired: 1 in, 2 out]
        n327 = Empty String/Path?(string/path=w626) -> (empty?=w625:bool)
        n328 = case shown="False" w625 {
          tunnel: [w641 _] -> w631
          tunnel: [w640 _] -> w630
          tunnel: w626 -> [w638 _]
          tunnel: w627 -> [w637 _]
          frame False {
            n329 = local read "Zoom Factor"() -> (w634:dbl)
            n330 = control-ref of="Preview"() -> (w636:refnum<vi>)
            n331 = Format Into String(format string="%s@%s", w637, w638) -> (resulting string=w640:string)  [unwired: 2 in, 1 out]
            n332 = call "Update Case Frame to Image.vi"("Zoom Factor"=w634, "Picture Control Reference"=w636, "Type"=enum16{"CSM", "CSM-VI"}."CSM-VI", "State"=w637, "Name"=w638) -> ("Error Out"=w641:errorcluster)  [unwired: 5 in, 1 out]
          }
          frame True {
          }
        }
        "StateInfo@Image" <- w630
      }
      frame "Action: Refresh Image" {
        n333 = control-ref of="CSM-States"() -> (w656:refnum<vi>)
        n334 = property class="LstBox (strict)"(reference=w656) -> ("Item Names"=w657:string[], "Value"=w655:i32[])  [unwired: 1 in, 2 out]
        n335 = control-ref of="MainTree"() -> (w653:refnum<vi>)
        n336 = property class="Tree (strict)"(reference=w653) -> ("Value"=w652:string[])  [unwired: 1 in, 2 out]
        n337 = Index Array(array=w655) -> (element=w654:i32)  [unwired: 1 in]
        n338 = Index Array(array=w652) -> (element=w651:string)  [unwired: 1 in]
        n339 = Match Pattern(string=w651, regular expression="/") -> (before substring=w645:string)  [unwired: 1 in, 3 out]
        n340 = Index Array(array=w657, index=w654) -> (element=w646:string)
        n341 = Concatenate Strings(w646, "@" ("string"), w645) -> (w643:string)
        n342 = call <vilib>:"Build State String with Arguments__JKI_lib_State_Machine.vi"("Arguments (\"\")"=w643, "State"="Action: Refresh Image API") -> ("State with Arguments"=w642:string)  [unwired: 4 in]
        n343 = call <vilib>:"Add State(s) to Queue__jki_lib_state_machine.vi"("State(s) in Front (\"\")"=w642, "State(s) in (\"\")"=w648) -> ("States Out"=w649:string)  [unwired: 13 in]
      }
      frame "Action: Refresh Image2" {
        n344 = control-ref of="CSM-Status"() -> (w663:refnum<vi>)
        n345 = property class="LstBox (strict)"(reference=w663) -> ("Item Names"=w677:string[], "Value"=w676:i32[])  [unwired: 1 in, 2 out]
        n346 = control-ref of="MainTree"() -> (w674:refnum<vi>)
        n347 = property class="Tree (strict)"(reference=w674) -> ("Value"=w673:string[])  [unwired: 1 in, 2 out]
        n348 = Index Array(array=w676) -> (element=w675:i32)  [unwired: 1 in]
        n349 = Index Array(array=w673) -> (element=w672:string)  [unwired: 1 in]
        n350 = Match Pattern(string=w672, regular expression="/") -> (before substring=w667:string)  [unwired: 1 in, 3 out]
        n351 = Index Array(array=w677, index=w675) -> (element=w661:string)
        n352 = Match Pattern(string=w661, regular expression="@") -> (after substring=w660:string)  [unwired: 1 in, 3 out]
        n353 = call <vilib>:"Trim Whitespace.vi"("string"=w660) -> ("trimmed string"=w659:string)  [unwired: 1 in]
        n354 = Concatenate Strings(w659, "@" ("string"), w667) -> (w665:string)
        n355 = call <vilib>:"Build State String with Arguments__JKI_lib_State_Machine.vi"("Arguments (\"\")"=w665, "State"="Action: Refresh Image API") -> ("State with Arguments"=w664:string)  [unwired: 4 in]
        n356 = call <vilib>:"Add State(s) to Queue__jki_lib_state_machine.vi"("State(s) in Front (\"\")"=w664, "State(s) in (\"\")"=w669) -> ("States Out"=w670:string)  [unwired: 13 in]
      }
      frame "Action: Refresh Symbol" {
        n357 = control-ref of="MainTree"() -> (w687:refnum<vi>)
        n358 = property class="Tree (strict)"(reference=w687) -> (reference out=w685:refnum<vi>, "All Tags"=w686:string[], "OwningVI"=w680:refnum<vi>)  [unwired: 1 in, 1 out]
        n359 = call "Defer Panel Updates_csm.vi"("Error In"=errorcluster {"status"=FALSE, "code"=0, "source"=""} ("error out"), "Defer Updates?"=TRUE, "VI Reference (Caller)"=w680) -> ("Error Out"=w683:errorcluster)  [unwired: 7 in, 1 out]
        n360 = for {
          tunnel: w686 -> [w692] mode=indexing
          tunnel: w685 -> [w693]
          shift-right: [w691] -> w679
          shift-left: w683 -> [w690]
          n361 = Match Pattern(string=w692, regular expression="/") -> (before substring=w694:string, offset past match=w696:i32)  [unwired: 1 in, 2 out]
          n362 = Less Than 0?(x=w696) -> (x < 0?=w695:bool)
          n363 = case shown="True" w695 {
            tunnel: w694 -> [_ w713]
            tunnel: w693 -> [w700 w714]
            tunnel: w692 -> [w699 w704]
            tunnel: [w701 w703] -> w691
            tunnel: w690 -> [w701 w702]
            frame False {
              n364 = property class="Tree (strict)"(reference=w700, "Active Item Tag"=w699, "Glyph"=18) -> ()  [unwired: 1 in, 2 out]
            }
            frame True {
              n365 = call "Read CSM-VI Info.vi"("CSM Name"=w713) -> ("Cluster 2"=w712:cluster{"Path":path})  [unwired: 9 in, 1 out]
              n366 = Unbundle By Name(w712) -> ("Path"=w711:path)
              n367 = Path To String(path=w711) -> (string=w710:string)
              n368 = call "lvcsm String to Path.vi"("Common Path"=w710) -> ("Path"=w709:path)  [unwired: 10 in]
              n369 = call "_VI Missing or Broken.vi"("Path"=w709) -> ("Missing Or Broken?"=w708:bool)  [unwired: 10 in]
              n370 = Select(t=2, s=w708, f=26) -> (s? t:f=w705:i32)
              n371 = property class="Tree (strict)"(reference=w714, error in=w702, "Active Item Tag"=w704, "Glyph"=w705) -> (error out=w703:errorcluster)  [unwired: 1 out]
            }
          }
        }
        n372 = call "Defer Panel Updates_csm.vi"("Error In"=w679, "Defer Updates?"=FALSE, "VI Reference (Caller)"=w680) -> ()  [unwired: 7 in, 2 out]
      }
      frame "Action: Change Zoom Factor" {
        n373 = Fract/Exp String To Number(string=w716) -> (number=w715:dbl)  [unwired: 3 in, 1 out]
        n374 = control-ref of="Preview"() -> (w717:refnum<vi>)
        n375 = property class="Pict"(reference=w717, "ZoomFactor"=w715) -> ()  [unwired: 1 in, 2 out]
      }
    }
  }
  n376 = while {
    shift-right: [w731] -> _
    shift-left: enum16{"Idle", "Initialize", "Exit"}."Initialize" -> [w732]
    tunnel: "Name (\"\" to Use Uuid)" -> [w729]
    shift-right: [w727] -> _
    shift-left: w12 -> [w728]
    shift-right: [w725] -> _
    shift-left: -1 -> [w726]
    shift-right: [w724] -> _
    shift-left: _ -> [w723]
    shift-right: [w722] -> _
    shift-left: _ -> [w721]
    stop <- w730 stop-if-true
    n377 = case shown="\"Initialize\"" w732 {
      tunnel: [enum16{"Idle", "Initialize", "Exit"}."Idle" w763 enum16{"Idle", "Initialize", "Exit"}."Exit"] -> w731
      tunnel: [_ _ TRUE] -> w730
      tunnel: w729 -> [w749 w762 _]
      tunnel: w728 -> [w752 w760 w938]
      tunnel: [w752 w761 w938] -> w727
      tunnel: w726 -> [_ w758 _]
      tunnel: [-1 w759 _] -> w725
      tunnel: [w748 w756 _] -> w724
      tunnel: w723 -> [_ w757 w937]
      tunnel: [w744 w754 w935] -> w722
      tunnel: w721 -> [_ w755 w935]
      frame "Initialize" {
        w737 = T11 {"Horizontal"=0, "Vertical"=0}  # PreviewMouseDownOrigin
        w738 = T11 {"Horizontal"=0, "Vertical"=0}  # PreviewMouseDownCoords
        w739 = FALSE  # PreviewMouseDown
        w745 = FALSE  # your data
        n378 = invoke class="VI" method="FP.Open"() -> (reference out=w741:refnum<vi>, error out=w742:errorcluster)  [unwired: 5 in, 3 out]
        n379 = call "CSM - Wait for Module to Be Alive.vi"("CSM Name"=w749) -> ("CSM Name (Dup)"=w747:string, "error out"=w746:errorcluster)  [unwired: 12 in, 1 out]
        n380 = call "Center Callee in Window Bounds.vi"("Error In"=w742, "Callee VI Refnum (Caller)"=w741, "Block Diagram Window:Window Bounds"="Caller Window Bounds") -> ("Error Out"=w743:errorcluster)  [unwired: 8 in]
        n381 = call "CSM - Module Exit Event.vi"("Error In"=w746, "Name (\"\" to Use UUID) In"=w747) -> ("CSM Exit Event"=w750:refnum<user-event>)  [unwired: 7 in, 2 out]
        n382 = call <vilib>:"Clear Errors.vi"("error in (no error)"=w743) -> ()  [unwired: 5 in, 2 out]
        n383 = register-events(w750) -> (reference out=w748:refnum<event-registration>)  [unwired: 2 in, 1 out]
        n384 = control-ref of="Interface-Filter"() -> (w733:refnum<vi>)
        n385 = control-ref of="Option:Sync Filter On States"() -> (w734:refnum<vi>)
        n386 = control-ref of="Zoom Factor"() -> (w735:refnum<vi>)
        n387 = Build Array(w733, w734, w735) -> (w736:refnum<vi>[])
        n388 = call "Distribute Controls Evenly.vi"("Controls"=w736) -> ()  [unwired: 10 in, 1 out]
        n389 = Bundle("your data"=w745, "PreviewMouseDown"=w739, "PreviewMouseDownCoords"=w738, "PreviewMouseDownOrigin"=w737) -> (w744:T12)  [unwired: 1 in]
      }
      frame "Idle", Default {
        n390 = event shown="[7] \"Preview\": Mouse Move" {
          selector: w757 -> [_ _ _ _ _ _ _ _ _ _ _ _ _ _ _ _ _ _ _ _ _ _ _ _ _ _ _ _]
          dyn-events: [_ _ _ _ _ _ _ _ _ _ _ _ _ _ _ _ _ _ _ _ _ _ _ _ _ _ _ _] -> w756
          timeout: w758 -> [_ _ _ _ _ _ _ _ _ _ _ _ _ _ _ _ _ _ _ _ _ _ _ _ _ _ _ _]
          tunnel: [_ enum16{"Idle", "Initialize", "Exit"}."Exit" enum16{"Idle", "Initialize", "Exit"}."Exit" _ _ _ _ _ _ _ _ _ _ _ _ _ _ _ _ _ _ _ _ _ _ _ _ _] -> w763
          tunnel: w762 -> [w765 w777 _ _ _ _ _ _ _ _ _ _ _ _ _ _ _ _ _ _ _ _ _ _ _ _ _ _]
          tunnel: w760 -> [w768 _ w782 w787 w790 w801 w805 w811 w819 w827 w830 w835 w839 w848 w853 w857 w861 w865 w876 w888 w896 w899 w901 w907 w912 w917 w927 w932]
          tunnel: [w766 w776 w782 w786 w791 w801 w805 w811 w820 w827 w831 w836 w840 w848 w854 w858 w862 w866 w876 w889 w896 w899 w902 w908 w913 w918 w927 w933] -> w761
          tunnel: [-1 _ _ 50 _ _ _ _ _ _ _ _ _ _ _ _ _ _ _ 20 _ _ 50 50 _ _ _ _] -> w759
          tunnel: w755 -> [w764 w775 w780 w783 w792 w794 w804 w810 w821 w826 w832 w837 w841 w847 w855 w859 w863 w867 w875 w892 w895 w898 w904 w910 w914 w919 w926 w934]
          tunnel: [w764 w775 w780 w783 w792 w793 w803 w810 w821 w826 w832 w837 w841 w847 w855 w859 w863 w867 w875 w892 w895 w898 w904 w910 w914 w919 w926 w934] -> w754
          event Timeout {
            n391 = event-data() -> ()  [unwired: 1 in, 3 out]
            n392 = call-poly "CSM - Filter JKISM String Queue.vi"("States In"=w768) -> ("States Out"=w767:string)  [unwired: 14 in]
            n393 = call "CSM - Forward UI Operations to CSM.vi"("Name (\"\" to Use UUID)"=w765, "State(s) In (\"\")"=w767) -> ("States Out"=w766:string)  [unwired: 8 in, 1 out]
          }
          event Panel Close? {
            n394 = event-data() -> ()  [unwired: 1 in, 1 out]
            n395 = call "CSM - Forward UI Operations to CSM.vi"("Name (\"\" to Use UUID)"=w777, "State(s) In (\"\")"="Macro: Exit" ("State")) -> ("States Out"=w776:string)  [unwired: 8 in, 1 out]
            n396 = Current VI's Path() -> (path=w774:path)
            n397 = Path To String(path=w774) -> (string=w773:string)
            n398 = Match Pattern(string=w773, regular expression="National Instruments") -> (offset past match=w771:i32)  [unwired: 1 in, 3 out]
            n399 = Less Than 0?(x=w771) -> (x < 0?=w770:bool)
            n400 = event-data("Discard?"=w770) -> ()  [unwired: 1 in, 1 out]
          }
          event User Event {
            n401 = event-data() -> ()  [unwired: 1 in, 1 out]
          }
          event Panel Resize {
            # "Wait 50ms to prevent flood of events"
            n402 = event-data() -> ()  [unwired: 1 in, 3 out]
            n403 = call <vilib>:"Add State(s) to Queue__JKI_lib_State_Machine.vi"("State(s) in (\"\")"=w787, "State(s) at Back (\"\")"="//Panel Size Message to CSM" ("State(s) at Back (\"\")")) -> ("States Out"=w786:string)  [unwired: 13 in]
          }
          event "MainTree": Value Change {
            n404 = event-data() -> ()  [unwired: 1 in, 1 out]
            n405 = call <vilib>:"Add State(s) to Queue__JKI_lib_State_Machine.vi"("State(s) in (\"\")"="Action: Refresh Interface\nAction: Refresh Status List" ("State")) -> ("States Out"=w789:string)  [unwired: 14 in]
            n406 = call <vilib>:"Add State(s) to Queue__JKI_lib_State_Machine.vi"("State(s) in Front (\"\")"=w789, "State(s) in (\"\")"=w790) -> ("States Out"=w791:string)  [unwired: 13 in]
          }
          event "Preview": Mouse Down {
            n407 = event-data() -> ("Button"=w795:u16, "CtlRef"=w796:refnum<vi>, "Coords"=w797:T11)  [unwired: 1 in, 2 out]
            n408 = property on="Property Node" class="Pict"(reference=w796) -> ("Origin"=w798:T5)  [unwired: 1 in, 2 out]
            n409 = Equal?(x=w795, y=u16 1) -> (x = y?=w800:bool)
            n410 = Bundle By Name(cluster=w794, "PreviewMouseDown"=w800, "PreviewMouseDownCoords"=w797, "PreviewMouseDownOrigin"=w798) -> (w793:T12)
          }
          event "Preview": Mouse Up {
            n411 = event-data() -> ()  [unwired: 1 in, 5 out]
            n412 = Bundle By Name(cluster=w804, "PreviewMouseDown"=FALSE) -> (w803:T12)
          }
          event "Preview": Mouse Move {
            n413 = event-data() -> ("Coords"=w806:T11)  [unwired: 1 in, 4 out]
            n414 = Unbundle By Name(w810) -> ("PreviewMouseDown"=w809:bool, "PreviewMouseDownCoords"=w808:T11, "PreviewMouseDownOrigin"=w807:T11)
            n415 = case shown="True" w809 {
              tunnel: w808 -> [_ w814]
              tunnel: w807 -> [_ w816]
              tunnel: w806 -> [_ w815]
              frame False {
              }
              frame True {
                n416 = Subtract(x=w815, y=w814) -> (x-y=w817:T11)
                n417 = Subtract(x=w816, y=w817) -> (x-y=w813:T11)
                n418 = control-ref of="Preview"() -> (w812:refnum<vi>)
                n419 = property on="Property Node" class="Pict"(reference=w812, "Origin"=w813) -> ()  [unwired: 1 in, 2 out]
              }
            }
          }
          event "Refresh", "Option:All-CSM-VIs", "Option:Online Only": Value Change {
            n420 = event-data() -> ()  [unwired: 1 in, 1 out]
            n421 = call <vilib>:"Add State(s) to Queue__JKI_lib_State_Machine.vi"("State(s) in Front (\"\")"="Macro: Refresh UI" ("Init State(\"Macro: Initialize\")"), "State(s) in (\"\")"=w819) -> ("States Out"=w820:string)  [unwired: 13 in]
          }
          event "MainTree": Shortcut Menu Activation? {
            n422 = event-data() -> ("CtlRef"=w822:refnum<vi>, "MenuRef"=w824:refnum<k9>, "Coords"=w823:T11)  [unwired: 1 in]
            n423 = call "Build MainTree Menu.vi"("CtlRef"=w822, "Coords"=w823, "Menu In"=w824) -> ("Discard?"=w825:bool)  [unwired: 8 in]
            n424 = event-data("Discard?"=w825) -> ()  [unwired: 1 in, 1 out]
          }
          event "MainTree": Shortcut Menu Selection (User) {
            n425 = event-data() -> ("ItemTag"=w828:string)  [unwired: 1 in, 7 out]
            n426 = case shown="Default" w828 {
              tunnel: [_ "Macro: Refresh UI" ("State(s) at Back (\"\")")] -> w829
              frame "COPY_CNT_FOLDER_TO_CLIPBOARD", "COPY_FULL_PATH_TO_CLIPBOARD", "EXPLORER_TO_FOLDER_ON_CSMVI", "OPEN_CSMVI_ON_CSM", "OPEN_CSMVI_ON_CSMVI" {
              }
              frame Default {
              }
            }
            n427 = call <vilib>:"Add State(s) to Queue__JKI_lib_State_Machine.vi"("State(s) in Front (\"\")"=w828, "State(s) in (\"\")"=w830, "State(s) at Back (\"\")"=w829) -> ("States Out"=w831:string)  [unwired: 12 in]
          }
          event "Interface-Filter": Value Change {
            n428 = event-data() -> ()  [unwired: 1 in, 6 out]
            n429 = call <vilib>:"Add State(s) to Queue__JKI_lib_State_Machine.vi"("State(s) in Front (\"\")"="Action: Refresh Interface" ("State(s) in Front (\"\")"), "State(s) in (\"\")"=w835) -> ("States Out"=w836:string)  [unwired: 13 in]
          }
          event "Open": Value Change {
            n430 = event-data() -> ()  [unwired: 1 in, 1 out]
            n431 = call <vilib>:"Add State(s) to Queue__JKI_lib_State_Machine.vi"("State(s) in Front (\"\")"="ADD_CSMVI_ON_MAINTREEE" ("Init State(\"Macro: Initialize\")"), "State(s) in (\"\")"=w839) -> ("States Out"=w840:string)  [unwired: 13 in]
          }
          event "CSM-States": Shortcut Menu Activation? {
            n432 = event-data() -> ("CtlRef"=w845:refnum<vi>, "MenuRef"=w846:refnum<k9>, "Coords"=w843:T11)  [unwired: 1 in, 4 out]
            n433 = control-ref of="MainTree"() -> (w842:refnum<vi>)
            n434 = call "Build Interface Menu.vi"("Tree"=w842, "CtlRef"=w845, "Coords"=w843, "Menu In"=w846) -> ("Discard?"=w844:bool)  [unwired: 7 in]
            n435 = event-data("Discard?"=w844) -> ()  [unwired: 1 in, 1 out]
          }
          event "CSM-States": Shortcut Menu Selection (User) {
            n436 = event-data() -> ("ItemTag"=w851:string)  [unwired: 1 in, 7 out]
            n437 = Match Pattern(string=w851, regular expression="#") -> (before substring=w849:string)  [unwired: 1 in, 3 out]
            n438 = call <vilib>:"Add State(s) to Queue__JKI_lib_State_Machine.vi"("State(s) in Front (\"\")"=w849, "State(s) in (\"\")"=w853, "State(s) at Back (\"\")"="" ("State(s) at Back (\"\")")) -> ("States Out"=w854:string)  [unwired: 12 in]
          }
          event "Scan Project": Value Change {
            n439 = event-data() -> ()  [unwired: 1 in, 5 out]
            n440 = call <vilib>:"Add State(s) to Queue__JKI_lib_State_Machine.vi"("State(s) in Front (\"\")"="SCAN_ALL_CSMVI\nMacro: Refresh UI" ("State(s) in Front (\"\")"), "State(s) in (\"\")"=w857) -> ("States Out"=w858:string)  [unwired: 13 in]
          }
          event "CSM-States": Double Click {
            n441 = event-data() -> ()  [unwired: 1 in, 5 out]
            n442 = call <vilib>:"Add State(s) to Queue__JKI_lib_State_Machine.vi"("State(s) in Front (\"\")"="Action: Refresh Image" ("State(s) in Front (\"\")"), "State(s) in (\"\")"=w861) -> ("States Out"=w862:string)  [unwired: 13 in]
          }
          event "CSM-Status": Double Click {
            n443 = event-data() -> ()  [unwired: 1 in, 5 out]
            n444 = call <vilib>:"Add State(s) to Queue__JKI_lib_State_Machine.vi"("State(s) in Front (\"\")"="Action: Refresh Image2" ("State(s) in Front (\"\")"), "State(s) in (\"\")"=w865) -> ("States Out"=w866:string)  [unwired: 13 in]
          }
          event "MainTree": Mouse Move {
            n445 = event-data() -> ("CtlRef"=w874:refnum<vi>, "Coords"=w873:T11)  [unwired: 1 in, 3 out]
            n446 = invoke class="Tree (strict)" method="Point To Row Column"(reference=w874, "Point"=w873) -> ("Tag"=w871:string)  [unwired: 6 in, 7 out]
            n447 = Match Pattern(string=w871, regular expression="/") -> (before substring=w869:string)  [unwired: 1 in, 3 out]
            n448 = feedback-in #1(w869) -> ()
            n449 = feedback #1() -> (w870:string)  [unwired: 1 in]
            n450 = Not Equal?(x=w869, y=w870) -> (x != y?=w868:bool)
            n451 = case shown="True" w868 {
              tunnel: w869 -> [_ w878]
              frame False {
              }
              frame True {
                n452 = call "Read CSM-VI Info.vi"("CSM Name"=w878) -> ("Cluster 2"=w884:cluster{"Path":path})  [unwired: 9 in, 1 out]
                n453 = Unbundle By Name(w884) -> ("Path"=w883:path)
                n454 = Path To String(path=w883) -> (string=w882:string)
                n455 = call "lvcsm String to Path.vi"("Common Path"=w882) -> ("Path"=w881:path)  [unwired: 10 in]
                n456 = Path To String(path=w881) -> (string=w880:string)
                n457 = Concatenate Strings(w878, "  ----  " ("string"), w880) -> (→"String":string)
              }
            }
          }
          event "Zoom Factor": Value Change {
            n458 = event-data() -> ()  [unwired: 1 in, 6 out]
            n459 = Number To Fractional String(number="Zoom Factor") -> (F-format string=w885:string)  [unwired: 3 in]
            n460 = call <vilib>:"Build State String with Arguments__JKI_lib_State_Machine.vi"("Arguments (\"\")"=w885, "State"="Action: Change Zoom Factor" ("State(s) in Front (\"\")")) -> ("State with Arguments"=w887:string)  [unwired: 4 in]
            n461 = call <vilib>:"Add State(s) to Queue__JKI_lib_State_Machine.vi"("State(s) in Front (\"\")"=w887, "State(s) in (\"\")"=w888) -> ("States Out"=w889:string)  [unwired: 13 in]
          }
          event "Zoom Factor", "Option:All-CSM-VIs", "Scan Project", "Preview", "Open", "Interface-Filter", "Play", "Fast Forward", "Fast Reverse", "Skip to Beginning", "Stop", "MainTree", "CSM-States": Mouse Enter {
            n462 = event-data() -> ("CtlRef"=w894:refnum<vi>)  [unwired: 1 in, 3 out]
            n463 = property class="Ctl"(reference=w894) -> ("TipStrip"=w893:string)  [unwired: 1 in, 2 out]
            n464 = local write "String"(w893) -> ()
          }
          event "MainTree", "CSM-States", "Interface-Filter", "Open", "Play", "Stop", "Skip to End", "Skip to Beginning", "Preview", "Fast Reverse", "Fast Forward", "Scan Project", "Option:All-CSM-VIs", "Zoom Factor": Mouse Leave {
            n465 = event-data() -> ()  [unwired: 1 in, 4 out]
            n466 = local write "String"("" ("String")) -> ()
          }
          event "Filter": Value Change {
            n467 = event-data() -> ()  [unwired: 1 in, 5 out]
            n468 = call <vilib>:"Add State(s) to Queue__JKI_lib_State_Machine.vi"("State(s) in Front (\"\")"="Action: Update Tree\nAction: Refresh Symbol" ("State(s) in Front (\"\")"), "State(s) in (\"\")"=w901) -> ("States Out"=w902:string)  [unwired: 13 in]
          }
          event "Reset Filter": Value Change {
            n469 = event-data() -> ()  [unwired: 1 in, 5 out]
            n470 = local write "Filter"("" ("Filter")) -> ()
            n471 = call <vilib>:"Add State(s) to Queue__JKI_lib_State_Machine.vi"("State(s) in Front (\"\")"="Action: Update Tree\nAction: Refresh Symbol" ("State(s) in Front (\"\")"), "State(s) in (\"\")"=w907) -> ("States Out"=w908:string)  [unwired: 13 in]
          }
          event "Refresh lvcsm Cache": Value Change {
            n472 = event-data() -> ()  [unwired: 1 in, 6 out]
            n473 = call <vilib>:"Add State(s) to Queue__JKI_lib_State_Machine.vi"("State(s) in Front (\"\")"="Action: Update Online CSMs\nAction: Refresh Symbol" ("State(s) in Front (\"\")"), "State(s) in (\"\")"=w912) -> ("States Out"=w913:string)  [unwired: 13 in]
          }
          event "Option:Sync Filter On States": Value Change {
            n474 = event-data() -> ()  [unwired: 1 in, 5 out]
            n475 = local read "FilterOption"() -> (w915:T2)
            n476 = case shown="\"State\"" w915 {
              tunnel: [_ "Action: Refresh Interface" ("Init State(\"Macro: Initialize\")")] -> w916
              frame "Name", Default {
              }
              frame "State" {
              }
            }
            n477 = call <vilib>:"Add State(s) to Queue__JKI_lib_State_Machine.vi"("State(s) in Front (\"\")"=w916, "State(s) in (\"\")"=w917) -> ("States Out"=w918:string)  [unwired: 13 in]
          }
          event "CSM-Status": Shortcut Menu Activation? {
            n478 = event-data() -> ("CtlRef"=w921:refnum<vi>, "MenuRef"=w924:refnum<k9>, "Coords"=w925:T11)  [unwired: 1 in, 4 out]
            n479 = control-ref of="MainTree"() -> (w922:refnum<vi>)
            n480 = call "Build Status Menu.vi"("Tree"=w922, "CtlRef"=w921, "Coords"=w925, "Menu In"=w924) -> ("Discard?"=w923:bool)  [unwired: 7 in]
            n481 = event-data("Discard?"=w923) -> ()  [unwired: 1 in, 1 out]
          }
          event "CSM-Status": Shortcut Menu Selection (User) {
            n482 = event-data() -> ("ItemTag"=w930:string)  [unwired: 1 in, 7 out]
            n483 = Match Pattern(string=w930, regular expression="#") -> (before substring=w928:string)  [unwired: 1 in, 3 out]
            n484 = call <vilib>:"Add State(s) to Queue__JKI_lib_State_Machine.vi"("State(s) in Front (\"\")"=w928, "State(s) in (\"\")"=w932, "State(s) at Back (\"\")"="" ("State(s) at Back (\"\")")) -> ("States Out"=w933:string)  [unwired: 12 in]
          }
        }
      }
      frame "Exit" {
        n485 = Unregister For Events(event registration refnum=w937) -> (error out=w936:errorcluster)  [unwired: 1 in]
        n486 = call <vilib>:"Clear Errors.vi"("error in (no error)"=w936) -> ()  [unwired: 5 in, 2 out]
      }
    }
  }
  n487 = control-ref of="Current VI Reference"() -> (w2:refnum<vi>)
  n488 = call "Close FP if in LabVIEW Dir.vi"("VI Refnum"=w2, "Error in"=w1) -> ("Error out"=w3:errorcluster)  [unwired: 9 in]
  n489 = call <vilib>:"Clear Errors.vi"("error in (no error)"=w3) -> ()  [unwired: 5 in, 2 out]
